vi "AlliGator Decay Actions.vi"(0 "AlliGator Q Elements in":T4[](array[typedef]), 1 "VI in":refnum<vi>, 2 "Script in":bool, 5 "AlliGator IV DVR in":refnum<data-value>, 7 "AlliGator Q Event in":T5=enum."GUI:Idle", 9 "Data":variant, 11 "error in (no error)":errorcluster, 12 "AlliGator Ctrl Refnums":T6) -> (3 "Script off":bool, 4 "AlliGator Q Elements out":T4[](array[typedef]), 6 "AlliGator IV DVR out":refnum<data-value>, 10 "[Notebook Message]":T1[](array[typedef]) {"Message Style"."Text Alignment" items=["Left", "Right", "Center"]}, 15 "error out":errorcluster)   [LabVIEW 2021, in "AlliGator Action Engine.lvlib"]
doc: "Processes AlliGator decay-related actions."
uses:
  AlliGator Action Engine.lvlib
  AlliGator Internal Variables v2.ctl
  <vilib>/vision/Image Controls.llb/IMAQ Image.ctl
  AlliGator Gate Image Set.ctl
  AlliGator FLI Dataset Type.ctl
  AlliGator Data Series Type.ctl
  AlliGator Dataset Channel.ctl
  AlliGator Gate Arithmetic.ctl
  AlliGator Displayed Image.ctl
  Image/Named ROI Description.ctl
  AlliGator Decay Metadata v3.ctl
  AlliGator Decay Background Subtraction Info.ctl
  AlliGator Baseline Subtraction Method.ctl
  Graphs/XY Graph/XY Graph Plot Shift Parameters.ctl
  Graphs/XY Graph/XY Graph Plot Shift Method.ctl
  AlliGator Decay Extrapolation Parameters.ctl
  Phasor/Calibration Phasor (m, phi).ctl
  Phasor/Phasor Reference Series.ctl
  Phasor/Phasor Calibration Map v2.ctl
  Phasor/Phasor (g, s).ctl
  AlliGator Raw Phasor Plot Data v4.ctl
  Phasor/Phasor Standard Deviation Options.ctl
  AlliGator Phasor Multi-Harmonic Data.ctl
  Phasor/Phasor Harmonic Data.ctl
  AlliGator Decay Fit Options & Parameters v2.ctl
  Fits/IRF(X)PSED/Decay Fit Options v2.ctl
  Fits/Decay Convolution/Decay Model.ctl
  Fits/Residual Type.ctl
  Fits/IRF(X)PSED/Fit Weights Type.ctl
  Fits/Non-linear Fitting Method v2.ctl
  Fits/Fit Calculation Method.ctl
  Fits/Non-linear Fitting Algorithm.ctl
  AlliGator Decay Fit Parameter Constraints 2.ctl
  Fits/IRF(X)PSED/Decay Fit Parameters In List.ctl
  Fits/IRF(X)PSED/MLE Baseline Offset Type.ctl
  AlliGator Decay Preprocessing Parameters.ctl
  Fits/IRF(X)PSED/Decay Fit Parameters & Derived Quantities List.ctl
  AlliGator Q Event.ctl
  AlliGator Ctrl Refnums.ctl
  AlliGator Other Ctrl Refnums.ctl
  AlliGator State Indicator.ctl
  AlliGator Phasor Plot Ctrl Refnums.ctl
  AlliGator Phasor Graph Ctrl Refnums.ctl
  Phasor/Phasor Calibration Type.ctl
  AlliGator Dataset Ctrl Refnums.ctl
  AlliGator Registered Events Ctrl Refnums.ctl
  AlliGator Image Histogram Control Refnums.ctl
  Histograms/Linear Histogram Options.ctl
  Histograms/Histogram Bin Option.ctl
  Histograms/Histogram Bin Position.ctl
  AlliGator Decay Fit Map Control Refnums.ctl
  AlliGator Q Element.ctl
  Notebook/Notebook Message Object.ctl
  Rich Text Box/Text Formatting.ctl
  Rich Text Box/Text Colors.ctl
  <vilib>/Utility/miscctls.llb/LVPoint32TypeDef.ctl
  Alligator Elements Order in Action Stack.ctl
  AlliGator State Indicators List.ctl
  AlliGator Settings List.ctl
  Graphs/XY Graph/XY Graph Selected Plot Info+Flag.ctl
  Graphs/XY Graph/XY Graph Refnum.ctl
  Fits/Square Pulse/Square Pulse Options.ctl
  Fits/Square Pulse/Square Pulse Levels Type.ctl
  Graphs/XY Graph/XY Graph Selected Plot Info.ctl
  Graphs/LabVIEW Plot Interpolation.ctl
  Variant/Variant to Data/Variant to I32.vi
  AlliGator Add Single Action to Stack.vi
  AlliGator Add Action Array to Stack.vi
  Variant/Variant to Data/Variant to U32.vi
  Variant/Variant to Data/Variant to DBL.vi
  GUI/GUI.lvlib
  AlliGator IRF.lvlib
  Variant/Variant to Data/Variant to Data.lvlib
  AlliGator GUI.lvlib
  AlliGator Decay Fit.lvlib
  Graphs/XY Graph/XY Graph Add-Ons.lvlib
  AlliGator Decay Processing.lvlib
  AlliGator Settings.lvlib
  Fits/Fits.lvlib
  AlliGator Internal Variables.lvlib
  AlliGator Decay Preprocessing.lvlib
  Graphs/Graphs.lvlib
  Sound/Sound.lvlib
  Fits/Abort Fit Global.vi
  AlliGator Intensity Corrections.lvlib
  Strings/Strings.lvlib
  Rich Text Box/Rich Text Box.lvlib
  Phasor/Phasor.lvlib
  Image/Image.lvlib
  AlliGator Phasor Graph.lvlib
  AlliGator Files.lvlib
  AlliGator Phasor Plot.lvlib
  AlliGator Source Image.lvlib
  AlliGator Decay Fit Parameter Map.lvlib
  AlliGator Dual-Channel Datasets.lvlib
  Histograms/Histogram Window.lvlib
  Notebook/Notebook.lvlib
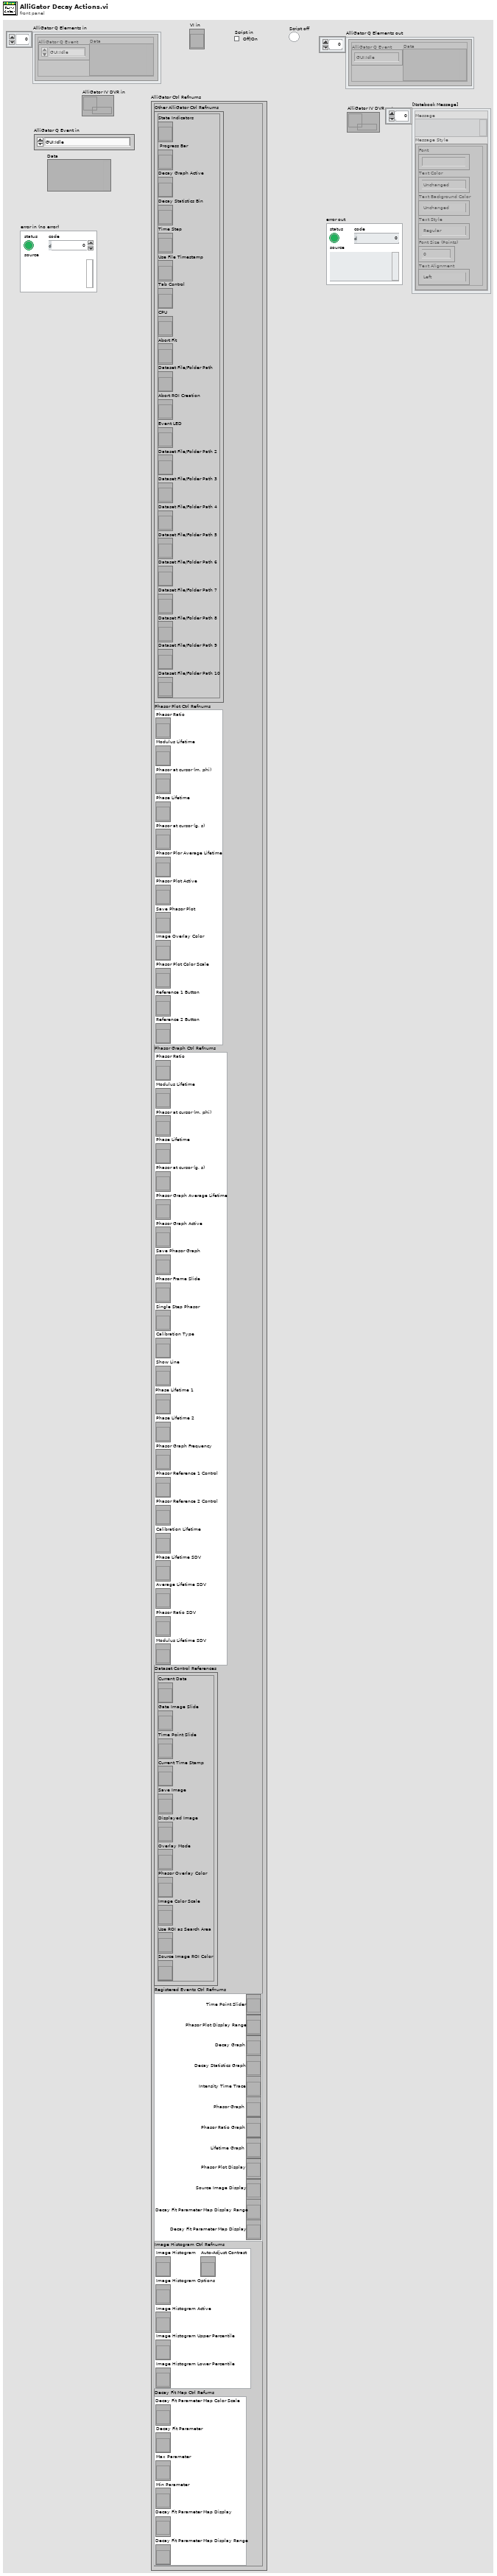
[diagram p1: front panel]
types:
  T1 = typedef "Notebook.lvlib/Notebook Message Object.ctl" = cluster{"Message":string, "Message Style":T2}
  T2 = typedef "Rich Text Box.lvlib/Text Formatting.ctl" = cluster{"Font":string, "Text Color":T3, "Text Background Color":T3, "Text Style":enum16{"Regular", "Bold", "Italic", "Underline", "Strikeout"}, "Font Size (Points)":dbl, "Text Alignment":i32}
  T3 = typedef "Rich Text Box.lvlib/Text Colors.ctl" = enum16{"Unchanged", "Black", "Blue", "Brown", "Gray", "Green", "Orange", "Pink", "Red", "White"}
  T4 = typedef "AlliGator Action Engine.lvlib/AlliGator Q Element.ctl" = cluster{"AlliGator Q Event":T5, "Data":variant}
  T5 = typedef "AlliGator Action Engine.lvlib/AlliGator Q Event.ctl" = enum16{"---- Files ----", "Files:Set Batch Export Files To Save", "Files:Set Dataset Loading & Pre-processing Options", "Files:Check #Frames in Dataset", "Files:Increment Frame Index", "Files:Open Mask Image", "Files:Open White Light Image", "Files:Open Single Dataset", "Files:New Folder of Folders Selected", "Files:Load File (all Types)_Scriptable", "Files:Move Flattened Series to Folders Series", "Files:Select Folder", "Files:Load FLI Dataset", "Files:Load Swiss SPAD 1 Dataset", "Files:Load Swiss SPAD 2 Dataset", "Files:Load .sdt FLI Dataset", "Files:Load .ptu FLI Dataset", "Files:Load .bin FLI Dataset", "Files:Load Single Gate Image Folder", "Files:Load I/m/phi Dataset (deprecated)", "Files:Load Single Image", "Files:Subtract Background File", "Files:Export FLI Dataset", "Files:Load HDF5 FLI Dataset", "Files:Set Destination File Path", "Files:Save Mask Image", "Files:Batch Conversion", "Files:New Folder Selected", "Files:Close FLI Dataset", "Files:Close FLI Dataset Series", "Files:Close White Light Image", "Files:Close Mask Image", "---- FLI Dataset ----", "FLI Dataset:Channel Arithmetic", "FLI Dataset:Export Average Lifetime Map as ASCII", "FLI Dataset:Export User-Defined Quantity Map as ASCII", "FLI Dataset:Python Function FLI Dataset Event", "FLI Dataset:ROI Analysis", "FLI Dataset:Tilted Logistic Square Gated IRF Characteristics Map", "FLI Dataset:Logistic Square Gated IRF Characteristics Map", "FLI Dataset:Square Gated IRF Characteristics Map", "FLI Dataset:Multi-ROI Single-Pixel Phasor Analysis", "FLI Dataset:Multi-ROI Single-Pixel NLSF Analysis", "FLI Dataset:All ROIs IRF Extraction", "FLI Dataset:All ROIs Decay Fit Non-Interactive (Fast + Individual IRF)", "FLI Dataset:All ROIs Phasor Analysis", "FLI Dataset:All ROIs Decay Fit", "FLI Dataset:Fluorescence Decay Statistics", "FLI Dataset:Update Decay Statistics Graph", "FLI Dataset:Get Decay from ROI", "FLI Dataset:All ROIs Average Lifetimes", "---- FLI Dataset Series ----", "FLI Dataset Series:Sum All Datasets in Series", "FLI Dataset Series:Add Dataset to Accumulated Dataset", "FLI Dataset Series:Display Accumulated Dataset", "FLI Dataset Series:Clear Dataset Series Sum", "FLI Dataset Series:Time-Series Analysis (NLSF)", "FLI Dataset Series:Time-Series Analysis (Phasor)", "---- Image ----", "Image:Update Image Profile Plots", "Image:Image Histogram Cursor Move", "Image:Image Histogram", "Image:Image Contrast", "Image:Set Image Histogram Cursor Move Flag", "Image:Clear Image Overlay", "Image:Use ROI as Search Area", "Image:Set ROI Diameter", "Image:Save Image Data as TIFF", "Image:Save Displayed Image with Overlay", "Image:Save Image Overlay Only", "Image:Save Image as Hot Pixel Mask", "Image:Change Source Image Color Palette", "Image:Copy Image to Clipboard", "Image:Source Image ROI Selection", "Image:Delete All ROIs", "Image:Delete All Unselected ROIs", "Image:Delete ROI", "Image:Merge All ROIs", "Image:Store ROI", "Image:Source Image ROI Storage", "Image:Export ROI Description to Notebook", "Image:Save ROI", "Image:Load ROI", "Image:Paste ROI Definition", "Image:Clear ROI", "Image:Identify ROIs in Mask Image", "Image:Create Complementary ROI", "Image:Create Contour ROI", "Image:Create ROI(s) from Pixels with Peak above Min_Scriptable", "Image:Create ROI(s) from Pixels with Intensity above Min_Scriptable", "Image:Compute ROI Statistics", "Image:Delete ROI(s) based on ROI Characteristics", "Image:Create ROI Grid", "Image:ROI to Individual Pixel ROIs", "Image:Python Function Source Image Event", "Image:Show Phasor Calibration Map ROI Centers", "Image:Convert ROI to Mask Image", "Image:Mouse Move", "Image:Mouse Up", "Image:Set Source Image Mouse Move Flag", "Image:Add Scale Bar Overlay", "Image:Delete Existing ROIs Option", "---- Decay ----", "Decay:Clear IRF/Reference Plot", "Decay:Clear Local IRFs", "Decay:Add Decay to Graph", "Decay:Smoothen Plot", "Decay:Smoothen Plot Tail", "Decay:Average Selected Plots", "Decay:Extract IRF", "Decay:Optimal IRF Extraction", "Decay:Threshold IRF", "Decay:Fit to Model IRF", "Decay:Fit IRF to Square Gate", "Decay:Fit IRF to Logistic Square Gate", "Decay:Fit IRF to Tilted Logistic Square Gate", "Decay:Create Bounding Cursors Set", "Decay:Export Bounding Cursors Definition to Notebook", "Decay:Denoise Plot", "Decay:Compute Cumulative Function", "Decay:Use as Reference Decay", "Decay:Show Reference Decay/IRF", "Decay:Extrapolate Decay", "Decay:Create Head & Tail Bounding Cursors", "Decay:Store Cursor-defined Head & Tail Fractions", "Decay:Rebin Plot", "Decay:1-Normalize Decay", "Decay:[0-1]-Normalize Plot", "Decay:Straighten Decay", "Decay:Shift Decay", "Decay:Fold Decay", "Decay:Fit Decay", "Decay:Global Fit of Selected Decays", "Decay:Post Global Fit Script", "Decay:Add Global Fit Parameters to Graph", "Decay:Add Decay Parameter(s) to Plot (Graph)", "Decay:Export Decay to Phasor Graph", "Decay:Plot Decay Shifts", "Decay:Compute Average Lifetime", "Decay:Plot Convolution", "Decay:Graph Tip Strip Update", "---- Decay Statistics ----", "Decay Statistics:Tip Strip Update", "---- Intensity Time Trace ----", "Intensity Time Trace:Use File Timestamp", "Intensity Time Trace:Load Intensity Corrections File", "Intensity Time Trace:Clear Intensity Corrections File", "Intensity Time Trace:Tip Strip Update", "---- Phasor Plot ----", "Phasor Plot:Build Phasor Plot", "Phasor Plot:Change Phasor Plot Color Palette", "Phasor Plot:Adjust Phasor Plot Display Range", "Phasor Plot:Highlight Image ROI in Phasor Plot", "Phasor Plot:Save Phasor Plot Image with Overlay", "Phasor Plot:Export Complex Phasor Map", "Phasor Plot:Export Phasor Ratio Map", "Phasor Plot:Export Average Lifetime Map", "Phasor Plot:Compute Phase Lifetime Histogram", "Phasor Plot:Compute Phasor Ratio Histogram", "Phasor Plot:Compute Phase Lifetime vs Intensity Scatter Plot", "Phasor Plot:Weber 2-Component Decomposition", "Phasor Plot:Update Phasor Color Map Vertices", "Phasor Plot:Clear Phasor Overlay", "Phasor Plot:Use Segment Extremities as References", "Phasor Plot:Use UC/Segment Intersections as References", "Phasor Plot:Use UC/Principal Axis Intersections as References", "Phasor Plot:Use UC/Linear Fit Intersections as References", "Phasor Plot:Update Phasor Plot Reference", "Phasor Plot:Show Local Phasor Info in Phasor Plot", "Phasor Plot:Update Phasor Plot State", "Phasor Plot:Phasor Plot ROI Storage", "Phasor Plot:Phasor Plot ROI Selection", "Phasor Plot:Python Function Phasor Plot Event", "Phasor Plot:Overlay Phasor ROI, Ratio or Map in Source Image", "Phasor Plot:Compute Decay of Selected Phasors", "Phasor Plot:Phasor at Image Pixel", "Phasor Plot:Mouse Move", "Phasor Plot:Mouse Up", "Phasor Plot:Display Range Mouse Move", "Phasor Plot:Set Mouse Move Flag", "---- Phasor Graph ----", "Phasor Graph:Calibrated Phasor Map Series", "Phasor Graph:Whole Image Phasor Scatter Plot (Todo)", "Phasor Graph:Get Phasor Value", "Phasor Graph:Create New Phasor Plot Dialog", "Phasor Graph:Update Last Phasor Value", "Phasor Graph:Update Phasor (m, phi)", "Phasor Graph:Remove Single Phasor from Plot", "Phasor Graph:Add Single Phasor to Plot", "Phasor Graph:Remove Phasor Plot", "Phasor Graph:Remove Selected Phasor Plots", "Phasor Graph:Clear Phasor Data", "Phasor Graph:Clear Phasor Graph", "Phasor Graph:Cursor Move", "Phasor Graph:Draw Cursor Connecting Line", "Phasor Graph:Clear Cursor Connecting Line", "Phasor Graph:Find UC Intersection", "Phasor Graph:Use UC/Cursor-Defined Line Intersections", "Phasor Graph:Use Selected Plots Fitted Line/UC Intersections", "Phasor Graph:Use Selected Plots Principal Axis/UC Intersections", "Phasor Graph:Show Single Phasor", "Phasor Graph:Save Single Phasor Plot", "Phasor Graph:Save All Phasor Plots", "Phasor Graph:Load Phasor Plot(s)", "Phasor Graph:Phasor Multiplication", "Phasor Graph:Compute Average Phasor", "Phasor Graph:Compute Multiple Average Phasors (Selected Plots)", "Phasor Graph:Export Single Phasor Plot Phase Lifetimes", "Phasor Graph:Phase Lifetime Trajectory", "Phasor Graph:Phase Lifetime vs Intensity Scatter Plot (deprecated)", "Phasor Graph:Parameter 2 vs Parameter 1 Scatter Plot", "Phasor Graph:Use Cursor n Location", "Phasor Graph:Set Reference n to Current Phase Lifetime Value", "Phasor Graph:Set Reference n to Lifetime Value", "Phasor Graph:Set Cursor n Location", "Phasor Graph:Save Phasor Graph Image", "Phasor Graph:Update SEPL Plot", "Phasor Graph:Export Single Phasor Plot Data", "Phasor Graph:Export Selected Phasor Plots Data", "Phasor Graph:Python Function Phasor Graph Event", "Phasor Graph:Tip Strip Update", "---- Calibration ----", "Calibration:Set Calibration Type", "Calibration:Load/Save Phasor Calibration", "Calibration:Load/Save Phasor Calibration Series", "Calibration:Load/Save Phasor Calibration Map", "Calibration:Use as Calibration", "Calibration:Compute Optimal Calibration from Phasor References", "Calibration:Clear Phasor Calibration", "Calibration:Single Phasor Calibration Information", "Calibration:Use as Calibration Series", "Calibration:Use as Calibration Map", "Calibration:Clear Calibration Series", "Calibration:Phasor Calibration Series Information", "Calibration:Clear Calibration Map", "Calibration:Phasor Calibration Map Information", "Calibration:Apply Phasor Calibration", "Calibration:Update Single Plot Calibration", "Calibration:Update Multiple Plots Calibration", "Calibration:Clear Single Plot Calibration", "Calibration:Clear All Plots Calibrations", "Calibration:Clear Plot(s) Calibration(s)?", "Calibration:Phasor Calibration Maps (# Gates Series)", "---- Phasor Ratio ----", "Phasor Ratio:Clear Reference n", "Phasor Ratio:Toggle Selected Plot(s)  Lock to Reference 1", "Phasor Ratio:Use as Reference n", "Phasor Ratio:Send Reference n to Notebook", "Phasor Ratio:Toggle Selected Plot(s)  Lock to Reference 2", "Phasor Ratio:Compute Phasor Ratio at Mouse Location", "Phasor Ratio:Compute Phasor Plot's Average Phasor Ratio", "Phasor Ratio:Compute Time-Series Phasor Ratios", "Phasor Ratio:Fit Line to Phasor Ratio Plot", "Phasor Ratio:Save References", "Phasor Ratio:Load References", "Phasor Ratio:Update Phasor Reference 1", "Phasor Ratio:Update Phasor Reference 2", "Phasor Ratio:Move Cursor n to Reference n", "Phasor Ratio:Use as Phasor Reference 1 Lifetime", "Phasor Ratio:Use as Phasor Reference 2 Lifetime", "Phasor Ratio:Export Phasor Ratio Map as ASCII", "Phasor Ratio:Tip Strip Update", "---- Lifetime & Other Parameters Graph ----", "Lifetime:Tip Strip Update", "---- Decay Fit Parameter Map ----", "Decay Fit Parameter Map:Export ROI NLSF Data as ASCII", "Decay Fit Parameter Map:Set Decay Fit  Parameter Map Selection", "Decay Fit Parameter Map:Build Decay Fit Parameter Map", "Decay Fit Parameter Map:Change Decay Fit Parameter Map Color Palette", "Decay Fit Parameter Map:Export Decay Fit Parameter Map Data as ASCII", "Decay Fit Parameter Map:Export All Decay Fit Parameter Maps Data as ASCII", "Decay Fit Parameter Map:Send Map Data to Lifetime Graph", "Decay Fit Parameter Map:Save Decay Fit Parameter Map Image", "Decay Fit Parameter Map:Save-Load IRFs & Fit Data", "Decay Fit Parameter Map:Update Local Decay Plots", "Decay Fit Parameter Map:Python Function Decay Fit Parameters Map Event", "Decay Fit Parameter Map:Overlay Decay Fit Parameter Map in Source Image", "Decay Fit Parameter Map:Plot Map Data vs Intensity", "Decay Fit Parameter Map:Mouse Up", "Decay Fit Parameter Map:Display Range Mouse Move", "---- Generic Graph ----", "Generic Graph:Generic XY Graph Event", "Generic Graph:Python Function XY Graph Event", "Generic Graph:New Plot", "Generic Graph:Save Plot", "Generic Graph:XY Plot Histogram", "Generic Graph:Set XY Graph Plot Name", "Generic Graph:Set Last Cursor Style", "Generic Graph:Tip Strip Update", "---- GUI ----", "GUI:Start Script", "GUI:Type of Displayed Image Changed", "GUI:Gate Image Slide Changed", "GUI:Show Busy Icon", "GUI:Show Busy Icon & Abort Button", "GUI:Hide Busy Icon", "GUI:Hide Busy Icon & Abort Button", "GUI:Abort", "GUI:End Script", "GUI:Start Timing", "GUI:End Timing", "GUI:Set State Indicator", "GUI:Send Parameters JSON Strings to Clipboard", "GUI:Set Gate Step", "GUI:Idle", "GUI:Initialization", "GUI:Quit", "GUI:Increment Dataset Index", "GUI:Set Dataset Index to -1", "GUI:Time Series Slider Moved", "GUI:Time Series Slider Changed", "GUI:Toggle Playback or Loop", "GUI:Playback Script", "GUI:Set Phasor Frequency", "GUI:Open Window", "GUI:Start Test Script", "GUI:End Test Script", "DEBUG"}
  T6 = typedef "AlliGator GUI.lvlib/AlliGator Ctrl Refnums.ctl" = cluster{"Other AlliGator Ctrl Refnums":T7, "Phasor Plot Ctrl Refnums":T8, "Phasor Graph Ctrl Refnums":T9, "Dataset Control References":T10, "Registered Events Ctrl Refnums":T11, "Image Histogram Ctrl Refnums":T12, "Decay Fit Map Ctrl Refums":T13}
  T7 = typedef "AlliGator GUI.lvlib/AlliGator Other Ctrl Refnums.ctl" = cluster{"State Indicators":refnum<vi>, " Progress Bar":refnum<vi>, "Decay Graph Active":refnum<vi>, "Decay Statistics Bin":refnum<vi>, "Time Step":refnum<vi>, "Use File Timestamp":refnum<vi>, "Tab Control":refnum<vi>, "CPU":refnum<vi>, "Abort Fit":refnum<vi>, "Dataset File/Folder Path":refnum<vi>, "Abort ROI Creation":refnum<vi>, "Event LED":refnum<vi>, "Dataset File/Folder Path 2":refnum<vi>, "Dataset File/Folder Path 3":refnum<vi>, "Dataset File/Folder Path 4":refnum<vi>, "Dataset File/Folder Path 5":refnum<vi>, "Dataset File/Folder Path 6":refnum<vi>, "Dataset File/Folder Path 7":refnum<vi>, "Dataset File/Folder Path 8":refnum<vi>, "Dataset File/Folder Path 9":refnum<vi>, "Dataset File/Folder Path 10":refnum<vi>}
  T8 = typedef "AlliGator GUI.lvlib/AlliGator Phasor Plot Ctrl Refnums.ctl" = cluster{"Phasor Ratio":refnum<vi>, "Modulus Lifetime":refnum<vi>, "Phasor at cursor (m, phi)":refnum<vi>, "Phase Lifetime":refnum<vi>, "Phasor at cursor (g, s)":refnum<vi>, "Phasor Plor Average Lifetime":refnum<vi>, "Phasor Plot Active":refnum<vi>, "Save Phasor Plot":refnum<vi>, "Image Overlay Color":refnum<vi>, "Phasor Plot Color Scale":refnum<vi>, "Reference 1 Button":refnum<vi>, "Reference 2 Button":refnum<vi>}
  T9 = typedef "AlliGator GUI.lvlib/AlliGator Phasor Graph Ctrl Refnums.ctl" = cluster{"Phasor Ratio":refnum<vi>, "Modulus Lifetime":refnum<vi>, "Phasor at cursor (m, phi)":refnum<vi>, "Phase Lifetime":refnum<vi>, "Phasor at cursor (g, s)":refnum<vi>, "Phasor Graph Average Lifetime":refnum<vi>, "Phasor Graph Active":refnum<vi>, "Save Phasor Graph":refnum<vi>, "Phasor Frame Slide":refnum<vi>, "Single Step Phasor":refnum<vi>, "Calibration Type":refnum<vi>, "Show Line":refnum<vi>, "Phase Lifetime 1":refnum<vi>, "Phase Lifetime 2":refnum<vi>, "Phasor Graph Frequency":refnum<vi>, "Phasor Reference 1 Control":refnum<vi>, "Phasor Reference 2 Control":refnum<vi>, "Calibration Lifetime":refnum<vi>, "Phase Lifetime SDV":refnum<vi>, "Average Lifetime SDV":refnum<vi>, "Phasor Ratio SDV":refnum<vi>, "Modulus Lifetime SDV":refnum<vi>}
  T10 = typedef "AlliGator GUI.lvlib/AlliGator Dataset Ctrl Refnums.ctl" = cluster{"Current Data":refnum<vi>, "Gate Image Slide":refnum<vi>, "Time Point Slide":refnum<vi>, "Current Time Stamp":refnum<vi>, "Save Image":refnum<vi>, "Displayed Image":refnum<vi>, "Overlay Mode":refnum<vi>, "Phasor Overlay Color":refnum<vi>, "Image Color Scale":refnum<vi>, "Use ROI as Search Area":refnum<vi>, "Source Image ROI Color":refnum<vi>}
  T11 = typedef "AlliGator GUI.lvlib/AlliGator Registered Events Ctrl Refnums.ctl" = cluster{"Time Point Slider":refnum<vi>, "Phasor Plot Display Range":refnum<vi>, "Decay Graph":refnum<vi>, "Decay Statistics Graph":refnum<vi>, "Intensity Time Trace":refnum<vi>, "Phasor Graph":refnum<vi>, "Phasor Ratio Graph":refnum<vi>, "Lifetime Graph":refnum<vi>, "Phasor Plot Display":refnum<vi>, "Source Image Display":refnum<vi>, "Decay Fit Parameter Map Display Range":refnum<vi>, "Decay Fit Parameter Map Display":refnum<vi>}
  T12 = typedef "AlliGator GUI.lvlib/AlliGator Image Histogram Control Refnums.ctl" = cluster{"Image Histogram":refnum<vi>, "Image Histogram Options":refnum<vi>, "Image Histogram Active":refnum<vi>, "Image Histogram Upper Percentile":refnum<vi>, "Image Histogram Lower Percentile":refnum<vi>, "Auto-Adjust Contrast":refnum<vi>}
  T13 = typedef "AlliGator Decay Fit Parameter Map.lvlib/AlliGator Decay Fit Map Control Refnums.ctl" = cluster{"Decay Fit Parameter Map Color Scale":refnum<vi>, "Decay Fit Parameter":refnum<vi>, "Max Parameter":refnum<vi>, "Min Parameter":refnum<vi>, "Decay Fit Parameter Map Display":refnum<vi>, "Decay Fit Parameter Map Display Range":refnum<vi>}
  T14 = typedef "AlliGator Action Engine.lvlib/Alligator Elements Order in Action Stack.ctl" = enum16{"Enqueue 2 AFTER 1", "Enqueue 2 BEFORE 1"}
  T15 = typedef "AlliGator Action Engine.lvlib/AlliGator State Indicators List.ctl" = enum16{"Phasor Calibration Defined", "Phasor Calibration Series Defined", "Phasor Calibration Map Defined", "Phasor Reference 1 Defined", "Phasor Reference 2 Defined", "Lifetime Reference 1 Defined", "Lifetime Reference 2 Defined", "Phasor Calibration Used", "Phasor Calibration Series Used", "Phasor Calibration Map Used", "Dataset Update Needed", "Phasor Plot Update Needed", "Reference/IRF Defined", "Individual IRFs Defined"}
  T16 = typedef "AlliGator Settings.lvlib/AlliGator Settings List.ctl" = enum16{"GUI:Visible Settings Tab", "GUI:Last Run Version", "Source Image:Use Image Histogram for Contrast", "Source Image:Low Count Pixels Rejection Options", "Source Image:High Count Pixels Rejection Options", "Source Image:Use Image Brightness", "Source Image:Blend Overlay with Image Background", "Source Image:Use Fixed ROI Diameter", "Source Image:ROI Diameter", "Source Image:ROI Center Color", "Source Image:Peak Threshold", "Source Image:Intensity Threshold", "Source Image:Image Binning Options", "Source Image:Image Smoothing Options", "Source Image:Image Histogram Active", "Source Image:Invert Binary Mask", "Source Image:Hot Pixel Removal", "Source Image:Overlay Analyzed ROI Center", "Source Image:Auto-Adjust Contrast", "Source Image:Histogram Lower Percentile", "Source Image:Histogram Upper Percentile", "Source Image:Save Source Image", "Source Image:Scale Bar Options", "Source Image:Image Resolution (Pixel Size)", "Source Image:Flatfield Correction", "Source Image:Show Dead Left Columns Correction", "Source Image:Dead Left Columns Correction", "Source Image:Image Pre-Processing Operations Order", "Data Information:Gate Width", "Data Information:Nanotime Gate Separation", "Data Information:Macrotime Gate Separation", "Data Information:Gate Step", "Data Information:# Gates", "Data Information:Gate Image Exposure", "Data Information:Gate Image Integration", "Data Information:Gates to Skip", "Data Information:Gates to Keep", "Data Information:Define Gates to", "Data Information:Channel Name", "Data Information:Available Channel Names", "Data Information:Channel Arithmetic", "Data Information:Background File Subtraction", "Data Information:Background File", "Data Information:Background Scaling Factor", "Data Information:Background Pile-up Correction", "Data Information:Background Pixel Well Capacity", "Data Information:Laser Period", "Data Information:SYNC Period", "Data Information:Pile-up Correction", "Data Information:Pixel Well Capacity", "Data Information:Dataset Scaling Factor", "Fluorescence Decay_Decay Pre-Processing:Reverse Gates", "Fluorescence Decay_Decay Pre-Processing:Verbose Decay Pre-Processing", "Fluorescence Decay_Decay Pre-Processing:Use Decay Pre-Processing", "Fluorescence Decay_Decay Pre-Processing:Background Subtraction", "Fluorescence Decay_Decay Pre-Processing:Background Definition Range", "Fluorescence Decay_Decay Pre-Processing:Baseline Subtraction Method", "Fluorescence Decay_Decay Pre-Processing:Decay Pre-Processing Operations Order", "Fluorescence Decay_Decay Pre-Processing:Smoothing Parameter", "Fluorescence Decay_Decay Pre-Processing:Shift Decay", "Fluorescence Decay_Decay Pre-Processing:Decay Shift Parameters", "Fluorescence Decay_Decay Pre-Processing:Fold Decay", "Fluorescence Decay_Decay Pre-Processing:# Folds", "Fluorescence Decay_Decay Pre-Processing:1-Normalize Decay", "Fluorescence Decay_Decay Pre-Processing:[0-1]-Normalize Decay", "Fluorescence Decay_Decay Pre-Processing:Smoothen Decay", "Fluorescence Decay_Decay Pre-Processing:Extrapolate Decay", "Fluorescence Decay_Decay Pre-Processing:Use Periodicity", "Fluorescence Decay_Decay Pre-Processing:Use Cursors", "Fluorescence Decay_Decay Pre-Processing:Tail Fraction", "Fluorescence Decay_Decay Pre-Processing:Head Fraction", "Fluorescence Decay_Decay Pre-Processing:Additional Points", "Fluorescence Decay_Decay Pre-Processing:Straighten Decay", "Fluorescence Decay_Decay Pre-Processing:Constant Background", "Fluorescence Decay_Decay Pre-Processing:Pixel-Normalize Decay", "Fluorescence Decay_Advanced Analysis:Extract IRF instead of Decay", "Fluorescence Decay_Advanced Analysis:IRF Extraction Options", "Fluorescence Decay_Advanced Analysis:IRF Optimization Options", "Fluorescence Decay_Advanced Analysis:Square Pulse Options", "Fluorescence Decay_Advanced Analysis:IRF Order", "Fluorescence Decay_Advanced Analysis:IRF Time Constants", "Fluorescence Decay_Advanced Analysis:Wavelet Analysis Options", "Fluorescence Decay_Advanced Analysis:Average Lifetime Options", "Fluorescence Decay_Fit Options:Fit Options", "Fluorescence Decay_Fit Options:Use Legacy Fitting Approach", "Fluorescence Decay_Fit Options:Use Data Information Laser Period", "Fluorescence Decay_Fit Parameters:Displayed Fit Parameters", "Fluorescence Decay_Fit Parameters:Fit Parameter Constraints", "Fluorescence Decay_Fit Parameters:Export Tabulated Results", "Fluorescence Decay_Fit Parameters:MLE Baseline Offset Type", "Fluorescence Decay_Fit Parameters:MLE Baseline Offset", "Fluorescence Decay_Fit Parameters:Guess Parameter Names", "Fluorescence Decay_Fit Parameters:Guess Parameter Values", "Fluorescence Decay_Fit Parameters:Guess Parameters Options", "Fluorescence Decay_Styles:Show Last Decay Only", "Fluorescence Decay_Styles:Decay Graph Color Array", "Fluorescence Decay:Decay Graph Active", "Fluorescence Decay Statistics:Min Peak Value", "Fluorescence Decay Statistics:Reject Low Decay Peak Pixels", "Fluorescence Decay Statistics:Reject High Decay Peak Pixels", "Fluorescence Decay Statistics:Max Peak Value", "Time Traces:Use File Timestamp", "Time Traces:Time Step", "Time Traces:Use Intensity Correction File", "Time Traces:Intensity Correction File", "Phasor Plot:Phasor Plot Smoothing Options", "Phasor Plot:Phasor Plot Size", "Phasor Plot:Phasor Plot Graphics Options", "Phasor Plot:Cumulative Phasor Plot", "Phasor Plot:Use Phasor Brightness", "Phasor Plot:Blend Overlay with Phasor Background", "Phasor Plot:Save Phasor Plot", "Phasor Plot:Show References", "Phasor Plot:Phasor Ratio Decay Range", "Phasor Plot:Exponential Fading", "Phasor Plot:Phasor Ratio Reference Colors", "Phasor Plot:Reference Radius", "Phasor Plot:Show Color Map Vertices", "Phasor Plot:Phasor Plot Active", "Phasor Plot:Phasor Ratio Color Map Type", "Phasor Plot:Phasor Ratio Color Map", "Phasor Plot:Phasor Ratio Display Range", "Phasor Plot:Selected Image ROI(s)", "Phasor Plot:All Image ROIs", "Phasor Plot:Selected Phasor Plot ROI(s)", "Phasor Plot:All Phasor Plot ROIs", "Phasor Plot:Phasor Ratio Color-Coded Quantity", "Phasor Plot:Store Phasor Harmonics", "Phasor Plot:Draw Reference Segment", "Phasor Plot:User-Defined Quantity", "Phasor Graph:Phasor Frequency", "Phasor Graph:Phasor Ratio Type", "Phasor Graph:Pixel-level Phasor Computation", "Phasor Graph:Save Phasor Graph", "Phasor Graph:Phasor Graph Active", "Phasor Graph:Phasor SDV Options", "Phasor Calibration:Use Backup Calibration if needed", "Phasor Graph:Define Shortest Lifetime as", "Phasor Calibration:Backup Calibration Type", "Phasor Calibration:Calibration Type", "Phasor Calibration:Calibration Lifetime", "Phasor Calibration:Calibration Map Algorithm", "Single-Exponential Phasor Locus (SEPL):Gate Parameters", "Single-Exponential Phasor Locus (SEPL):User-defined Gate", "Single-Exponential Phasor Locus (SEPL):User-defined IRF", "Single-Exponential Phasor Locus (SEPL):Phasor Parameters", "Single-Exponential Phasor Locus (SEPL):Decay & IRF Parameters", "Single-Exponential Phasor Locus (SEPL):Display Parameters", "Lifetime Analysis:Decay Analysis Parameters", "Lifetime Analysis:Lifetime Map Active", "Plugins:Python Settings", "Miscellaneous:Verbose Mode", "Miscellaneous:Beep after Script", "Miscellaneous:Saved Image File Format", "Miscellaneous:Exported Gate Image Settings", "Miscellaneous:Include Loading in Timing", "Miscellaneous:Verbose Settings Mode", "Miscellaneous:Histogram Options", "Miscellaneous:Beep on Error", "Miscellaneous:# Logical Processors Used", "Miscellaneous:ROI Description Max Characters", "Miscellaneous:Verbose Error Mode", "Miscellaneous:Transparent Mask Color"}
  T17 = typedef "XY Graph Add-Ons.lvlib/XY Graph Selected Plot Info+Flag.ctl" = cluster{"Multiplot XY Graph":T18, "Mouse Coordinates":T19, "Plot Index":i32, "Flag":bool}
  T18 = typedef "XY Graph Add-Ons.lvlib/XY Graph Refnum.ctl" = refnum<vi>
  T19 = typedef "LVPoint32TypeDef.ctl" = cluster{"Horizontal":i32, "Vertical":i32}
  T20 = typedef "Fits.lvlib/Square Pulse Options.ctl" = cluster{"Method":T21, "# Bins":i32, "Threshold %":dbl, "Center on Midpoint":bool, "Smoothen Plot":bool}
  T21 = typedef "Fits.lvlib/Square Pulse Levels Type.ctl" = enum16{"Mode", "Mean"}
  T22 = typedef "XY Graph Add-Ons.lvlib/XY Graph Selected Plot Info.ctl" = cluster{"Multiplot XY Graph":T18, "Mouse Coordinates":T19, "Plot Index":i32}
  T23 = typedef "AlliGator Decay Analysis.lvlib/AlliGator Decay Fit.lvlib/AlliGator Decay Fit Output Options.ctl" = cluster{"Fit Model":T24, "Decay Fit Parameter Array":T25[]}
  T24 = typedef "Fits.lvlib/Decay Model.ctl" = enum16{"1-Exponential", "2-Exponentials"}
  T25 = typedef "Fits.lvlib/Decay Fit Parameters & Derived Quantities List.ctl" = enum16{"Offset", "Baseline", "A_1", "tau_1", "A_2", "tau_2", "<tau>_a", "f1_a", "f2_a", "<tau>_i", "f1_i", "f2_i", "-", "R^2", "Chi^2"}
  T26 = cluster{"CtlRef":refnum<vi>, "Coords":T19, "Plot ID":i32}
  T27 = typedef "Math.lvlib/Wavelet Analysis Options.ctl" = cluster{"Wavelet":enum16{"db02", "db03", "db04", "db05", "db06", "db07", "db08", "db09", "db10", "db11", "db12", "db13", "db14", "Haar", "bior1_3", "bior1_5", "bior2_2", "bior2_4", "bior2_6", "bior2_8", "bior3_1", "bior3_3", "bior3_5", "bior3_7", "bior3_9", "bior4_4 (FBI)", "bior5_5", "bior6_8", "coif1", "coif2", "coif3", "coif4", "coif5", "sym2", "sym3", "sym4", "sym5", "sym6", "sym7", "sym8"}, "Option for Approximate Coefficients":enum16{"None", "Threshold", "Detrend"}, "# Levels":i32, "Threshold Settings":cluster{"Thresholding Rule":enum16{"SURE", "Hybrid", "Universal", "Minimax"}, "Rescaling Method":enum16{"One", "Single level", "Multiple levels"}, "Soft Threshold?":bool}, "Wavelet Transform Type":enum16{"Discrete", "Undecimated"}}
  T28 = typedef "ROI Descriptor" = cluster{"Global Rectangle":i32[], "Contours":cluster{"ID":enum32{"External", "Internal"}, "Type":u32, "Coordinates":i32[]}[]}
  T29 = typedef "XY Graph Add-Ons.lvlib/XY Plot Data.ctl" = cluster{"X Array":dbl[], "Y Array":dbl[]}
  T30 = typedef "AlliGator Decay Fit Parameter Map.lvlib/AlliGator Decay Fit Options & Parameters v2.ctl" = cluster{"SYNC Period":dbl[unit], "Fit Options":T31, "Fit Parameter Constraints":T37[], "MLE Baseline Offset":dbl, "MLE Baseline Offset Type":T39}
  T31 = typedef "Fits.lvlib/Decay Fit Options v2.ctl" = cluster{"Show Fit Residuals":bool, "Fit Model":T24, "Residual Type":T32, "Max Decay Percentile":dbl, "Min Decay Percentile":dbl, "Show Full Decay":bool, "Weights":T33, "Fitting Method":T34, "Compute Parameter Uncertainties":bool, "Periodic Boundaries":bool, "Model Calculation":T35, "Period":dbl[unit], "Termination Criteria":cluster{"Max Iterations":i32, "Max Function Calls":i32, "Max Time":dbl[unit], "Function Tolerance":dbl, "Parameter Tolerance":dbl, "Gradient Tolerance":dbl, "Min Lambda":dbl, "Max Lambda":dbl, "Initial Tick Count":u32}, "Offset Resolution":dbl[unit], "Use Local IRF":bool, "Fitting Algorithm":T36}
  T32 = typedef "Fits.lvlib/Residual Type.ctl" = enum16{"Standard", "Normalized", "Reduced"}
  T33 = typedef "Fits.lvlib/Fit Weights Type.ctl" = enum16{"Unweighted", "1/Variance", "Best of All"}
  T34 = typedef "Fits.lvlib/Non-linear Fitting Method v2.ctl" = enum16{"Least Square", "Least Absolute Residual", "Bisquare", "MLE", "-", "Best of All"}
  T35 = typedef "Fits.lvlib/Fit Calculation Method.ctl" = enum16{"Simulation", "Convolution", "Integration"}
  T36 = typedef "Fits.lvlib/Non-linear Fitting Algorithm.ctl" = enum16{"Levenberg-Marquardt", "Trust-Region Dogleg"}
  T37 = typedef "AlliGator Decay Analysis.lvlib/AlliGator Decay Fit.lvlib/AlliGator Decay Fit Parameter Constraints 2.ctl" = cluster{"Fit Parameter":T38, "Min Value":dbl, "Max Value":dbl, "Global":bool, "Used":bool}
  T38 = typedef "Fits.lvlib/Decay Fit Parameters In List.ctl" = enum16{"Offset", "Baseline", "A_1", "tau_1", "A_2", "tau_2"}
  T39 = typedef "Fits.lvlib/MLE Baseline Offset Type.ctl" = enum32{"Absolute", "Percentage"}
  T40 = cluster{"t Array":dbl[], "Amplitude Array":dbl[]}
  T41 = typedef "XY Graph Add-Ons.lvlib/XY Graph Plot Shift Parameters.ctl" = cluster{"Type":T42, "Shift":dbl[unit], "Threshold":dbl, "Rotate":bool}
  T42 = typedef "XY Graph Add-Ons.lvlib/XY Graph Plot Shift Method.ctl" = enum16{"Default", "CFD", "Threshold", "Cross-Correlation"}
  T43 = typedef "Graphs.lvlib/LabVIEW Plot Interpolation.ctl" = u8
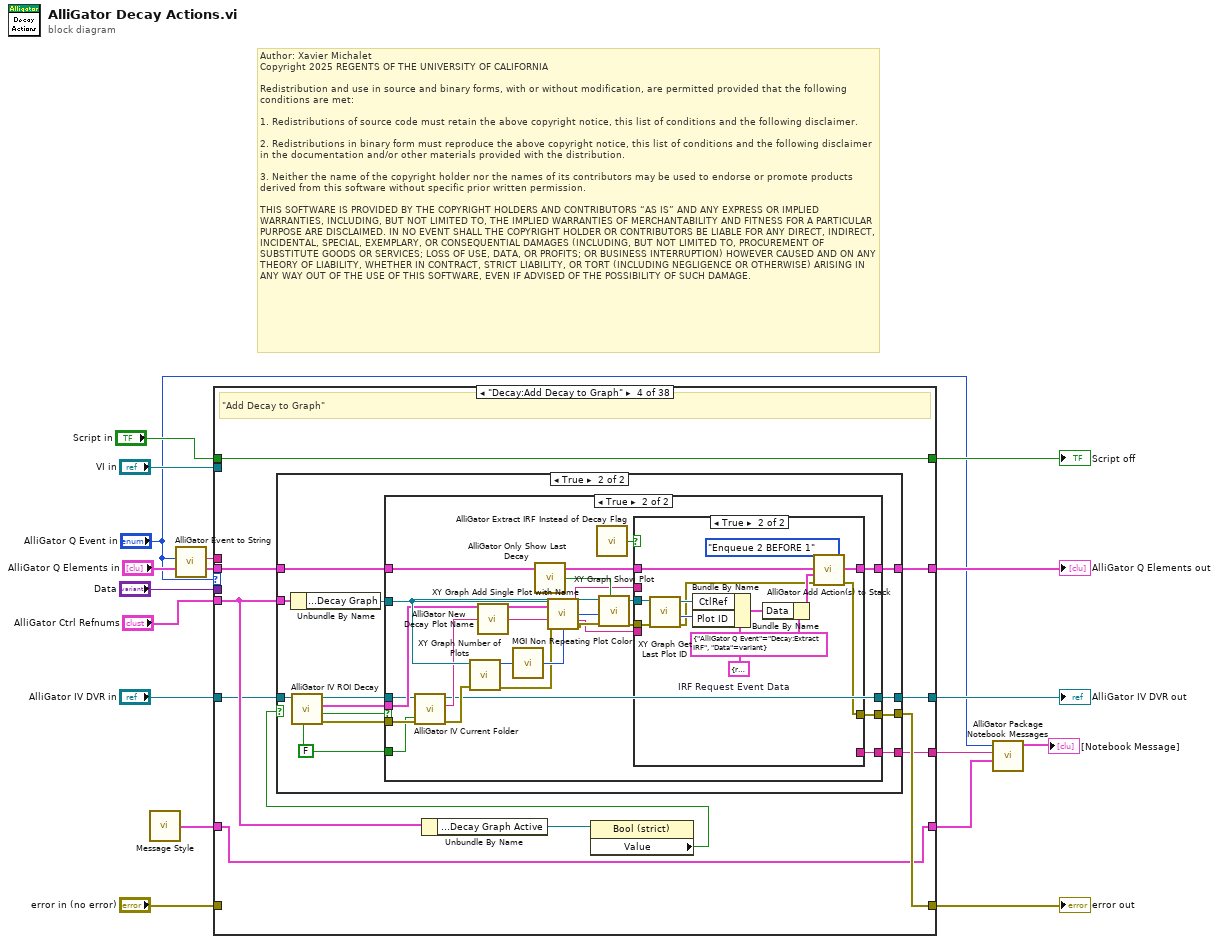
[diagram p0: block diagram]
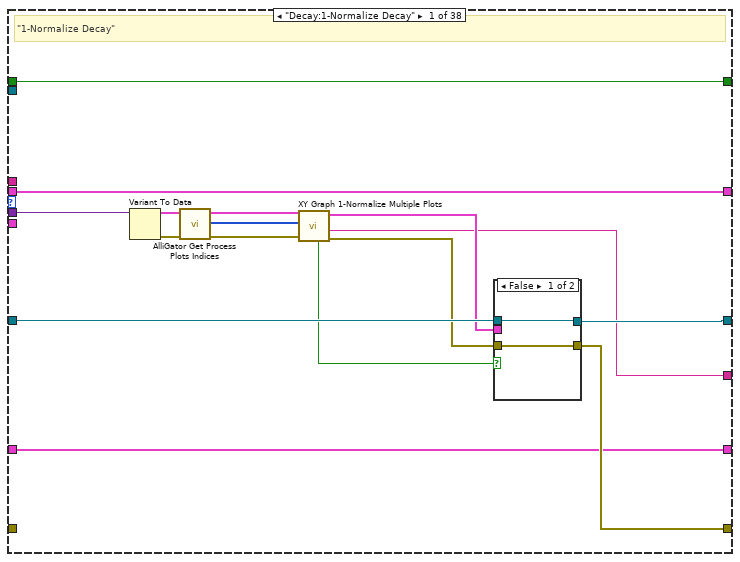
[diagram p2: hidden frame]
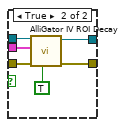
[diagram p3: hidden frame]
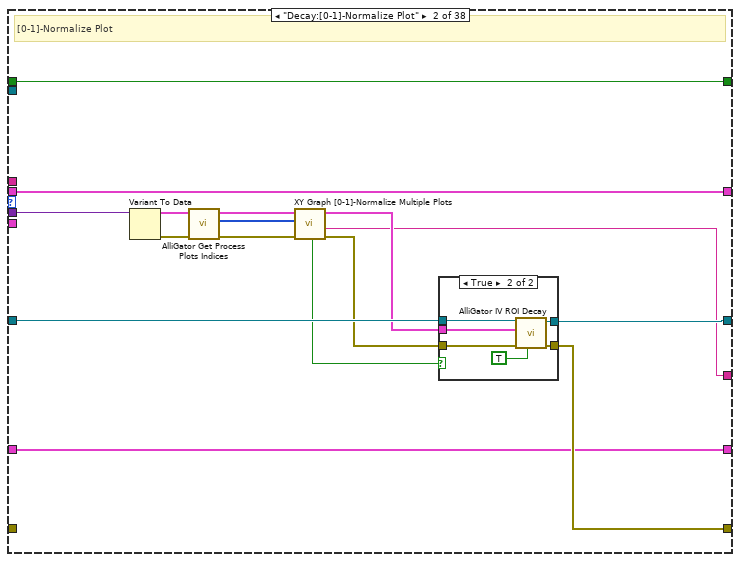
[diagram p4: hidden frame]
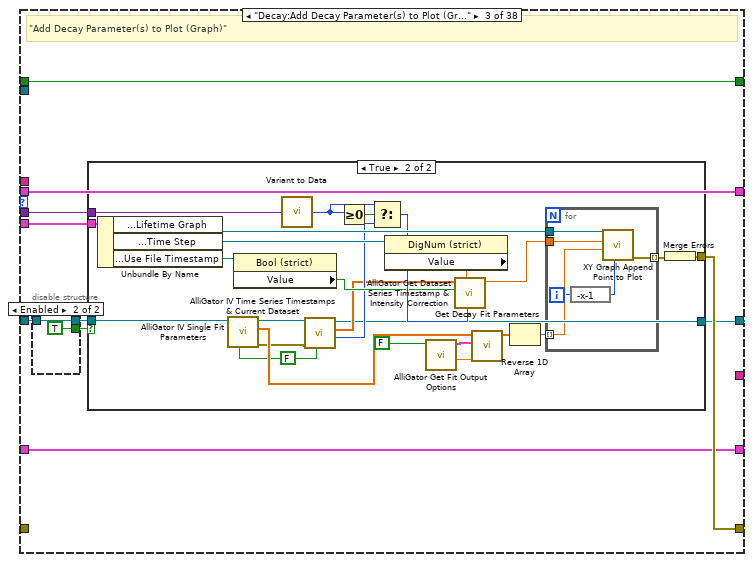
[diagram p6: hidden frame]
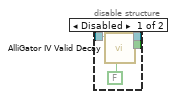
[diagram p7: hidden frame]
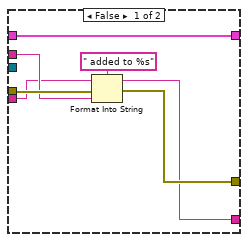
[diagram p11: hidden frame]
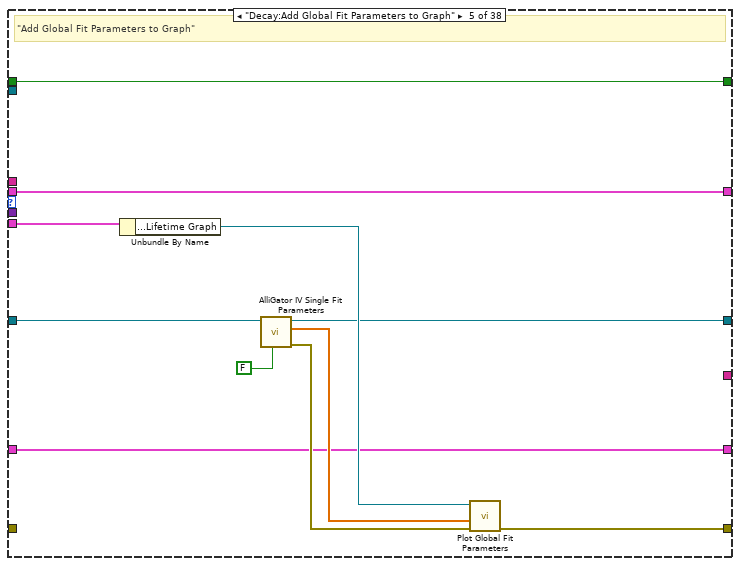
[diagram p12: hidden frame]
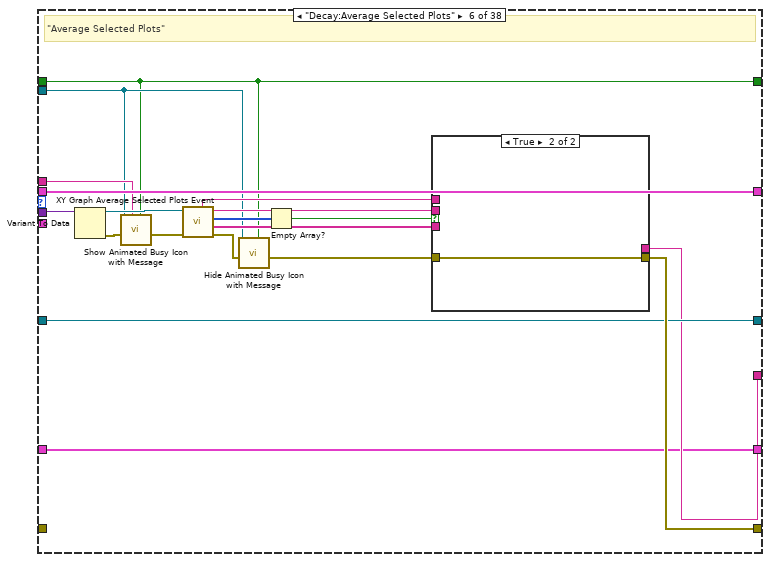
[diagram p13: hidden frame]
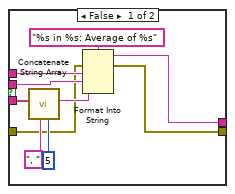
[diagram p14: hidden frame]
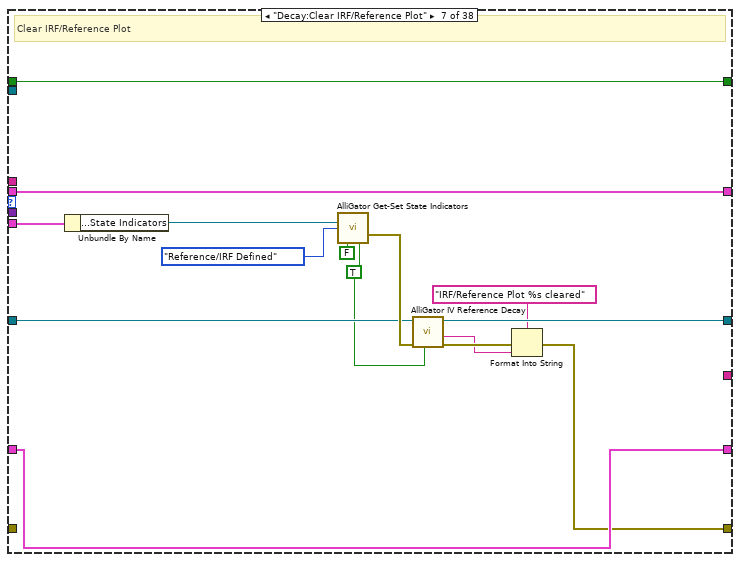
[diagram p15: hidden frame]
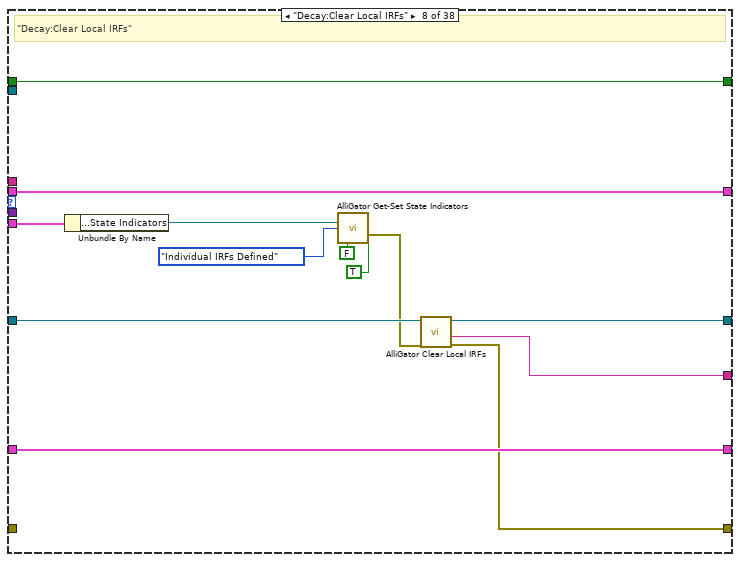
[diagram p16: hidden frame]
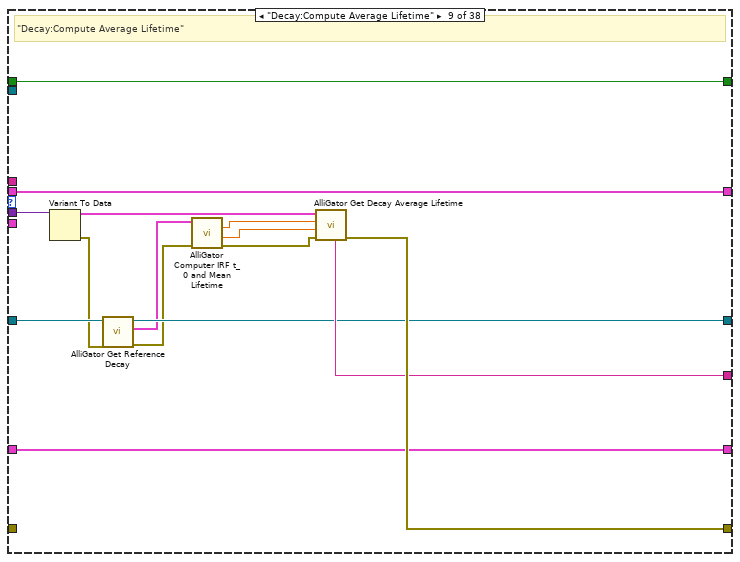
[diagram p17: hidden frame]
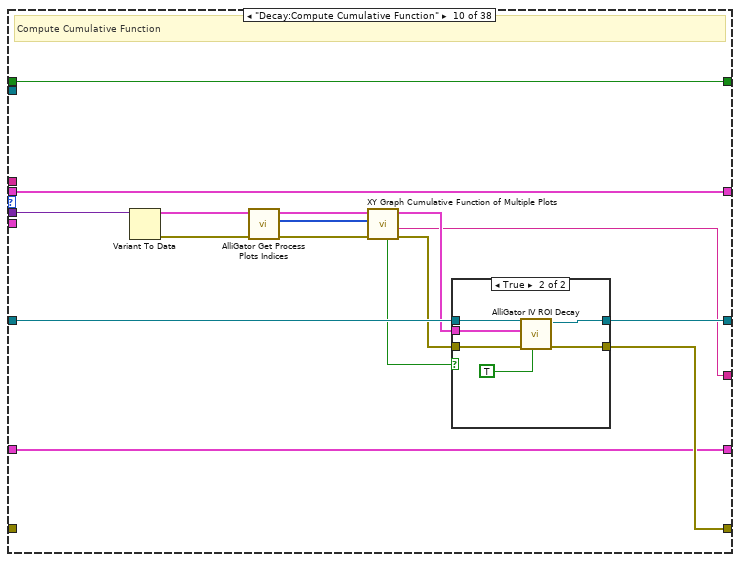
[diagram p18: hidden frame]
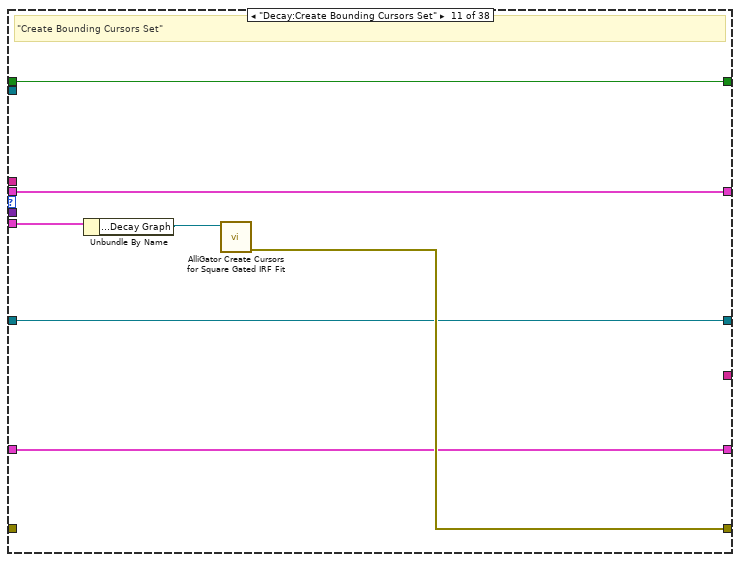
[diagram p20: hidden frame]
diagram:
  # "Author: Xavier Michalet\nCopyright 2025 REGENTS OF THE UNIVERSITY OF CALIFORNIA\n\nRedistribution and use in source and binary forms, with or without modification, are permitted provided that the following conditions are met:\n\n1. Redistributions of source code must retain the above copyright notice, this list of conditions and the following disclaimer.\n\n2. Redistributions in binary form must reproduce the above copyright notice, this list of conditions and the following disclaimer in the documentation and/or other materials provided with the distribution.\n\n3. Neither the name of the copyright holder nor the names of its contributors may be used to endorse or promote products derived from this software without specific prior written permission.\n\nTHIS SOFTWARE IS PROVIDED BY THE COPYRIGHT HOLDERS AND CONTRIBUTORS “AS IS” AND ANY EXPRESS OR IMPLIED WARRANTIES, INCLUDING, BUT NOT LIMITED TO, THE IMPLIED WARRANTIES OF MERCHANTABILITY AND FITNESS FOR A PARTICULAR PURPOSE ARE DISCLAIMED. IN NO EVENT SHALL THE COPYRIGHT HOLDER OR CONTRIBUTORS BE LIABLE FOR ANY DIRECT, INDIRECT, INCIDENTAL, SPECIAL, EXEMPLARY, OR CONSEQUENTIAL DAMAGES (INCLUDING, BUT NOT LIMITED TO, PROCUREMENT OF SUBSTITUTE GOODS OR SERVICES; LOSS OF USE, DATA, OR PROFITS; OR BUSINESS INTERRUPTION) HOWEVER CAUSED AND ON ANY THEORY OF LIABILITY, WHETHER IN CONTRACT, STRICT LIABILITY, OR TORT (INCLUDING NEGLIGENCE OR OTHERWISE) ARISING IN ANY WAY OUT OF THE USE OF THIS SOFTWARE, EVEN IF ADVISED OF THE POSSIBILITY OF SUCH DAMAGE."
  n1 = call "Message Style.vi"() -> ("Message Formatting"=w5:T2)
  n2 = call "AlliGator Event to String.vi"("AlliGator Q Event"="AlliGator Q Event in") -> ("String"=w8:string)  [unwired: 8 in]
  n3 = case shown="\"Decay:Add Decay to Graph\"" "AlliGator Q Event in" {
    selector: "AlliGator Q Event in" -> [_ _ _ _ _ _ _ _ _ _ _ _ _ _ _ _ _ _ _ _ _ _ _ _ _ w678 _ _ _ _ _ _ _ _ _ _ w918 _]
    tunnel: "Data" -> [w32 w56 w72 _ _ w217 _ _ w268 w286 _ _ w330 _ w351 w400 w416 w436 w478 w515 w532 w549 w568 _ w656 w680 _ _ w731 w766 _ w815 w844 w859 w877 w898 w920 _]
    tunnel: "AlliGator Q Elements in" -> [w33 w57 w75 w125 w198 w216 w243 w256 w271 w287 w302 w309 w331 w350 w361 w401 w417 w437 w484 w516 w533 w550 w569 w587 w657 w681 w705 w713 w732 w767 w787 w816 w845 w862 w878 w899 w921 w926]
    tunnel: [w33 w57 w75 w124 w198 w216 w243 w256 w271 w287 w302 w309 w331 w350 w360 w401 w417 w437 w484 w516 w533 w550 w569 w586 w657 w681 w705 w712 w732 w767 w787 w816 w845 w862 w878 w899 w921 w926] -> w10
    tunnel: "VI in" -> [_ _ _ _ _ w203 _ _ _ _ _ _ _ _ _ w394 _ w432 w486 w504 w528 w545 _ w583 w650 _ _ _ _ _ _ _ _ _ _ _ _ _]
    tunnel: [w30 w54 w74 w123 w197 w199 w242 w255 w270 w284 w301 w308 w322 w342 w362 w385 w414 w434 w476 w493 w517 w534 w567 w585 w641 w676 w700 w716 w729 w765 w786 w810 w839 w861 w875 w896 w916 w925] -> w7
    tunnel: "Script in" -> [w30 w54 w74 w123 w197 w199 w242 w255 w270 w284 w301 w308 w322 w342 w362 w385 w414 w434 w476 w493 w517 w534 w567 w585 w641 w676 w700 w716 w729 w765 w786 w810 w839 w861 w875 w896 w916 w925]
    tunnel: w8 -> [_ _ _ _ _ w204 _ _ _ _ _ _ _ _ _ w395 _ w433 w485 w503 w527 w544 _ w582 w651 _ _ _ _ _ _ _ _ _ _ _ _ _]
    tunnel: "error in (no error)" -> [_ _ _ _ _ _ _ _ _ _ _ _ _ _ _ _ _ _ _ _ _ _ _ _ _ _ _ _ _ _ _ _ _ _ _ _ _ w924]
    tunnel: [w26 w50 w73 w122 w196 w205 w231 w245 w269 w279 w300 w307 w319 w345 w359 w390 w409 w435 w481 w498 w523 w539 w561 w588 w646 w677 w701 w709 w724 w762 w785 w806 w835 w860 w870 w891 w917 w924] -> w6
    tunnel: "AlliGator Ctrl Refnums" -> [_ _ w71 w120 w194 _ w241 w254 _ _ w298 w305 _ w344 w357 _ _ _ _ _ _ _ _ w584 _ _ w698 w714 _ _ w780 _ _ _ _ _ w914 _]
    tunnel: "AlliGator IV DVR in" -> [w28 w52 w67 w118 w193 w202 w235 w248 w262 w283 w297 w304 w317 w343 w355 w393 w413 w427 w483 w501 w525 w543 w563 w581 w649 w673 w696 w707 w727 w761 w779 w809 w838 w857 w874 w895 w912 w923]
    tunnel: [w29 w53 w70 w117 w189 w202 w234 w247 w261 w282 w297 w304 w318 w343 w354 w392 w412 w431 w482 w502 w526 w542 w559 w580 w648 w671 w697 w707 w728 w763 w777 w808 w837 w857 w873 w894 w913 w923] -> w17
    tunnel: [w20 w44 _ w115 _ w201 _ w244 w263 w278 _ _ w316 w341 w353 w387 w408 w430 w480 w496 w520 w537 w558 w579 w643 w675 w692 _ w723 w757 _ w804 w833 w856 w869 w889 w907 _] -> w3
    tunnel: [w25 w49 w69 w116 w188 w200 w240 w253 w267 w277 w296 w303 w315 w340 w352 w386 w407 w429 w479 w495 w519 w536 w557 w578 w642 w674 w691 w706 w722 w756 w776 w803 w832 w855 w868 w888 w906 w922] -> w2
    tunnel: w5 -> [w25 w49 w69 w116 w188 w200 w240 w253 w267 w277 w296 w303 w315 w340 w352 w386 w407 w429 w479 w495 w519 w536 w557 w578 _ w674 w691 w706 w722 w756 w776 w803 w832 w855 w868 w888 w906 w922]
    frame "Decay:1-Normalize Decay" {
      # "\"1-Normalize Decay\""
      n4 = Variant To Data(Variant=w32) -> (data=w24:T22, error out=w31:errorcluster)  [unwired: 2 in]
      n5 = call "AlliGator Get Process Plots Indices.vi"("error in (no error)"=w31, "Selected Plot Info"=w24) -> ("error out"=w22:errorcluster, "Selected Plots"=w18:i32[], "Selected Plot Info (dup)"=w23:T22)  [unwired: 7 in]
      n6 = call "XY Graph 1-Normalize Multiple Plots.vi"("error in (no error)"=w22, "Selected Plots"=w18, "Selected Plot Info"=w23) -> ("error out"=w27:errorcluster, "1-Normalize Plot Message"=w20:string, "Last 1-Normalized Plot"=w21:cluster{"t Array":dbl[], "IRF Array":dbl[]}, "Single Plot?"=w19:bool)  [unwired: 5 in]
      n7 = case shown="False" w19 {
        tunnel: [w35 w41] -> w29
        tunnel: w28 -> [w35 w40]
        tunnel: w27 -> [w34 w39]
        tunnel: [w34 w38] -> w26
        tunnel: w21 -> [_ w36]
        frame False {
        }
        frame True {
          n8 = call "AlliGator IV ROI Decay.vi"("Get (F)/ Set (T)"=TRUE, "error in (no error)"=w39, "Decay in"=w36, "AlliGator IV DVR in"=w40) -> ("error out"=w38:errorcluster, "AlliGator IV DVR out"=w41:refnum<data-value>)  [unwired: 4 in, 2 out]
        }
      }
    }
    frame "Decay:[0-1]-Normalize Plot" {
      # "[0-1]-Normalize Plot"
      n9 = Variant To Data(Variant=w56) -> (data=w47:T22, error out=w55:errorcluster)  [unwired: 2 in]
      n10 = call "AlliGator Get Process Plots Indices.vi"("error in (no error)"=w55, "Selected Plot Info"=w47) -> ("error out"=w48:errorcluster, "Selected Plots"=w42:i32[], "Selected Plot Info (dup)"=w46:T22)  [unwired: 7 in]
      n11 = call "XY Graph [0-1]-Normalize Multiple Plots.vi"("error in (no error)"=w48, "Selected Plots"=w42, "Selected Plot Info"=w46) -> ("error out"=w51:errorcluster, "[0-1]-Normalize Plot Message"=w44:string, "Last [0-1]-Normalized Plot"=w45:cluster{"t Array":dbl[], "IRF Array":dbl[]}, "Single Plot?"=w43:bool)  [unwired: 5 in]
      n12 = case shown="True" w43 {
        tunnel: [w59 w65] -> w53
        tunnel: w52 -> [w59 w64]
        tunnel: w51 -> [w58 w63]
        tunnel: [w58 w62] -> w50
        tunnel: w45 -> [_ w61]
        frame False {
        }
        frame True {
          n13 = call "AlliGator IV ROI Decay.vi"("Get (F)/ Set (T)"=TRUE, "error in (no error)"=w63, "Decay in"=w61, "AlliGator IV DVR in"=w64) -> ("error out"=w62:errorcluster, "AlliGator IV DVR out"=w65:refnum<data-value>)  [unwired: 4 in, 2 out]
        }
      }
    }
    frame "Decay:Add Decay Parameter(s) to Plot (Graph)" {
      # "\"Add Decay Parameter(s) to Plot (Graph)\""
      n14 = disable-structure shown="Enabled" {
        disable-tunnel: [w78 w81] -> w68
        disable-tunnel: w67 -> [w77 w81]
        disable-tunnel: [w76 TRUE ("Valid Decay")] -> w66
        frame Disabled {
          n15 = call "AlliGator IV Valid Decay.vi"("Get (F)/ Set (T)"=FALSE, "AlliGator IV DVR in"=w77) -> ("Valid Decay"=w76:bool, "AlliGator IV DVR out"=w78:refnum<data-value>)  [unwired: 7 in, 1 out]
        }
        frame Enabled {
        }
      }
      n16 = case shown="True" w66 {
        tunnel: [_ w104] -> w73
        tunnel: w72 -> [_ w102]
        tunnel: w71 -> [_ w95]
        tunnel: [w82 w85] -> w70
        tunnel: w68 -> [w82 w83]
        frame False {
        }
        frame True {
          w84 = FALSE ("Get (F)/ Set (T)")
          n17 = Unbundle By Name(w95) -> ("Registered Events Ctrl Refnums.Lifetime Graph"=w103:refnum<vi>, "Other AlliGator Ctrl Refnums.Time Step"=w94:refnum<vi>, "Other AlliGator Ctrl Refnums.Use File Timestamp"=w92:refnum<vi>)
          n18 = call "AlliGator IV Single Fit Parameters.vi"("Get (F)/ Set (T)"=w84, "AlliGator IV DVR in"=w83) -> ("error out"=w87:errorcluster, "[Single Decay Fit Parameter]"=w90:dbl[], "AlliGator IV DVR out"=w89:refnum<data-value>)  [unwired: 7 in]
          n19 = property class="Bool (strict)"(reference=w92) -> ("Value"=w91:bool)  [unwired: 1 in, 2 out]
          n20 = call-poly "Variant to Data.vi"("Variant"=w102) -> ("Value"=w100:i32)  [unwired: 8 in]
          n21 = call "AlliGator IV Time Series Timestamps & Current Dataset.vi"("Get (F)/ Set"=w84, "error in (no error)"=w87, "AlliGator IV DVR in"=w89) -> ("Current Dataset"=w88:i32, "[Time-Series Timestamps]"=w86:dbl[], "AlliGator IV DVR out"=w85:refnum<data-value>)  [unwired: 5 in, 1 out]
          n22 = Greater Or Equal To 0?(x=w100) -> (x >= 0?=w101:bool)
          n23 = Select(t=w100, s=w101, f=w88) -> (s? t:f=w99:i32)
          n24 = property class="DigNum (strict)"(reference=w94) -> ("Value"=w93:dbl[unit])  [unwired: 1 in, 2 out]
          n25 = call "AlliGator Get Fit Output Options.vi"("All Parameters?"=FALSE) -> ("Laser Period"=w96:dbl, "Decay Fit Output Options"=w98:T23)  [unwired: 8 in, 1 out]
          n26 = call "AlliGator Get Dataset Series Timestamp & Intensity Correction.vi"("Current Data Set"=w99, "Time Step"=w93, "Use File Timestamp"=w91, "Dataset Series Timestamps"=w86) -> ("Time Stamp (s)"=w108:dbl)  [unwired: 6 in, 1 out]
          n27 = call "Get Decay Fit Parameters.vi"("Laser Period"=w96, "Decay Fit Output Options"=w98, "Decay Fit Parameters"=w90) -> ("Displayed Decay Fits Parameters"=w107:dbl[])  [unwired: 7 in, 1 out]
          n28 = Reverse 1D Array(array=w107) -> (reversed array=w106:dbl[])
          n29 = for {
            tunnel: w103 -> [w114]
            tunnel: w108 -> [w113]
            tunnel: w106 -> [w112] mode=indexing
            tunnel: [w109] -> w105 mode=indexing
            i -> [w111]
            n30 = expression code="-x-1"(w111) -> (w110:i32)
            n31 = call "XY Graph Append Point to Plot.vi"("Plot ID (-1: last)"=w110, "y"=w112, "x"=w113, "XYGraph in"=w114) -> ("error out"=w109:errorcluster)  [unwired: 4 in, 3 out]
          }
          n32 = Merge Errors(w105) -> (w104:errorcluster)
        }
      }
    }
    frame "Decay:Add Decay to Graph" {
      # "\"Add Decay to Graph\""
      n33 = Unbundle By Name(w120) -> ("Other AlliGator Ctrl Refnums.Decay Graph Active"=w121:refnum<vi>)
      n34 = property class="Bool (strict)"(reference=w121) -> ("Value"=w119:bool)  [unwired: 1 in, 2 out]
      n35 = case shown="True" w119 {
        tunnel: w125 -> [w127 w140]
        tunnel: [w127 w139] -> w124
        tunnel: w120 -> [_ w138]
        tunnel: [_ w136] -> w122
        tunnel: w118 -> [w126 w135]
        tunnel: [w126 w130] -> w117
        tunnel: [_ w129] -> w115
        frame False {
        }
        frame True {
          w131 = FALSE ("Get (F)/ Set (T)")
          n36 = Unbundle By Name(w138) -> ("Registered Events Ctrl Refnums.Decay Graph"=w137:refnum<vi>)
          n37 = call "AlliGator IV ROI Decay.vi"("Get (F)/ Set (T)"=w131, "AlliGator IV DVR in"=w135) -> ("error out"=w132:errorcluster, "Valid Decay?"=w128:bool, "Decay out"=w134:cluster{"t Array":dbl[], "IRF Array":dbl[]}, "AlliGator IV DVR out"=w133:refnum<data-value>)  [unwired: 6 in]
          n38 = case shown="True" w128 {
            tunnel: w140 -> [w143 w167]
            tunnel: [w143 w166] -> w139
            tunnel: w137 -> [_ w156]
            tunnel: [w141 w154] -> w136
            tunnel: w134 -> [_ w153]
            tunnel: w133 -> [w142 w152]
            tunnel: w132 -> [w141 w151]
            tunnel: w131 -> [_ w149]
            tunnel: [w142 w147] -> w130
            tunnel: [_ w144] -> w129
            frame False {
            }
            frame True {
              n39 = call "AlliGator IV Current Folder.vi"("Get (F)/ Set (T)"=w149, "error in (no error)"=w151, "AlliGator IV DVR in"=w152) -> ("error out"=w148:errorcluster, "Current Folder"=w150:string, "AlliGator IV DVR out"=w147:refnum<data-value>)  [unwired: 6 in]
              n40 = call "XY Graph Number of Plots.vi"("Error In"=w148, "XYGraph in"=w156) -> ("Error Out"=w155:errorcluster, "# Plots"=w157:i32)  [unwired: 8 in]
              n41 = call "AlliGator New Decay Plot Name.vi"("Current Folder"=w150) -> ("New Decay Name"=w164:string)  [unwired: 8 in]
              n42 = call <userlib>:"MGI Non Repeating Plot Color.vi"("Plot #"=w157) -> ("Color"=w158:u32)
              n43 = call "AlliGator Only Show Last Decay.vi"() -> ("Show Last Decay Only?"=w161:bool)
              n44 = call "XY Graph Add Single Plot with Name.vi"("XYGraph Ref in"=w156, "Plot"=w153, "Plot Name (\"Plot\")"=w164, "error in (no error)"=w155, "Plot Color (Default)"=w158) -> ("XY Graph Caption (or Label)"=w145:string, "Plot Index"=w162:i32, "Plot Name"=w146:string, "error out"=w163:errorcluster)  [unwired: 7 in]
              n45 = call "AlliGator Extract IRF Instead of Decay Flag.vi"() -> ("Extract IRF instead of Decay?"=w165:bool)
              n46 = call "XY Graph Show Plot.vi"("Hide All Other Plots (F)"=w161, "error in (no error)"=w163, "Selected Plot Index"=w162, "XYGraph in"=w156) -> ("error out"=w159:errorcluster, "XYGraph out"=w160:T18)  [unwired: 6 in]
              n47 = case shown="True" w165 {
                tunnel: w160 -> [_ w182]
                tunnel: w167 -> [w174 w180]
                tunnel: [w174 w177] -> w166
                tunnel: w159 -> [w173 w181]
                tunnel: [w172 w175] -> w154
                tunnel: w146 -> [w168 _]
                tunnel: w145 -> [w171 _]
                tunnel: [w169 _] -> w144
                frame False {
                  n48 = Format Into String(format string=" added to %s", initial string=w168, error in=w173, w171) -> (resulting string=w169:string, error out=w172:errorcluster)
                }
                frame True {
                  w183 = T26 {"CtlRef"=refnum, "Coords"={"Horizontal"=0, "Vertical"=0}, "Plot ID"=0}  # IRF Request Event Data
                  n49 = call "XY Graph Get Last Plot ID.vi"("error in (no error)"=w181, "XYGraph in"=w182) -> ("error out"=w178:errorcluster, "Last Plot ID"=w184:i32, "XYGraph out"=w185:refnum<vi>)  [unwired: 7 in]
                  n50 = Bundle By Name(cluster=w183, "CtlRef"=w185, "Plot ID"=w184) -> (w186:T26)
                  n51 = Bundle By Name(cluster=T4 {"AlliGator Q Event"=enum."Decay:Extract IRF", "Data"=variant} ("element"), "Data"=w186) -> (w179:T4)
                  n52 = call-poly "AlliGator Add Action(s) to Stack.vi"("Elements Order in Action Stack (Default: 2 BEFORE 1)"=Alligator_Elements_Order_in_Action_Stack."Enqueue 2 BEFORE 1", "Error In"=w178, "Alligator Atomic Action"=w179, "Alligator Queue Element 1"=w180) -> ("Error Out"=w175:errorcluster, "Alligator Queue Element 1 (+ 2)"=w177:T4[])  [unwired: 6 in]
                }
              }
            }
          }
        }
      }
    }
    frame "Decay:Add Global Fit Parameters to Graph" {
      # "\"Add Global Fit Parameters to Graph\""
      n53 = Unbundle By Name(w194) -> ("Registered Events Ctrl Refnums.Lifetime Graph"=w195:refnum<vi>)
      n54 = call "AlliGator IV Single Fit Parameters.vi"("Get (F)/ Set (T)"=FALSE, "AlliGator IV DVR in"=w193) -> ("error out"=w191:errorcluster, "[Single Decay Fit Parameter]"=w192:dbl[], "AlliGator IV DVR out"=w189:refnum<data-value>)  [unwired: 7 in]
      n55 = call "Plot Global Fit Parameters.vi"("Error In"=w191, "Best Fit Parameters"=w192, "XYGraph in"=w195) -> ("Error Out"=w196:errorcluster)  [unwired: 8 in]
    }
    frame "Decay:Average Selected Plots" {
      # "\"Average Selected Plots\""
      n56 = Variant To Data(Variant=w217) -> (data=w212:refnum<vi>, error out=w209:errorcluster)  [unwired: 2 in]
      n57 = call "Show Animated Busy Icon with Message.vi"("Already active? (F)"=w199, "Message"=w204, "Error In"=w209, "Target VI Refnum"=w203) -> ("Error Out"=w211:errorcluster)  [unwired: 7 in]
      n58 = call "XY Graph Average Selected Plots Event.vi"("Error In"=w211, "XYGraph Ref"=w212) -> ("Error Out"=w210:errorcluster, "Averaged Plot Names"=w215:string[], "Averaged Plot Indices"=w214:i32[], "Graph Label"=w208:string, "Plot Name"=w207:string)  [unwired: 5 in]
      n59 = call "Hide Animated Busy Icon with Message.vi"("Already active? (F)"=w199, "Error In"=w210, "Target VI reference"=w203) -> ("Error Out"=w206:errorcluster)  [unwired: 8 in]
      n60 = Empty Array?(array=w214) -> (empty?=w213:bool)
      n61 = case shown="True" w213 {
        tunnel: w215 -> [w225 _]
        tunnel: w208 -> [w226 _]
        tunnel: w207 -> [w222 _]
        tunnel: w206 -> [w219 w228]
        tunnel: [w221 w228] -> w205
        tunnel: [w218 _] -> w201
        frame False {
          n62 = call "Concatenate String Array.vi"("Max Number of Elements (None: -1)"=5 ("Max Number of Elements (None: 1)"), "Separator (TAB)"=", ", "String Array"=w225) -> ("Formatted String"=w223:string)  [unwired: 8 in]
          n63 = Format Into String(format string="%s in %s: Average of %s", error in=w219, w222, w226, w223) -> (resulting string=w218:string, error out=w221:errorcluster)  [unwired: 1 in]
        }
        frame True {
        }
      }
    }
    frame "Decay:Clear IRF/Reference Plot" {
      w232 = TRUE ("Set (T)/Get")
      # "Clear IRF/Reference Plot"
      n64 = Unbundle By Name(w241) -> ("Other AlliGator Ctrl Refnums.State Indicators"=w237:refnum<vi>)
      n65 = call "AlliGator Get-Set State Indicators.vi"("State Indicators Refnum"=w237, "AlliGator State Indicators List"=AlliGator_State_Indicators_List."Reference/IRF Defined", "ON/OFF"=FALSE, "Set (T)/Get"=w232) -> ("Error Out"=w236:errorcluster)  [unwired: 9 in, 2 out]
      n66 = call "AlliGator IV Reference Decay.vi"("Get (F)/ Set (T)"=w232, "Error In"=w236, "AlliGator IV DVR in"=w235) -> ("Error Out"=w233:errorcluster, "Reference Decay Plot Name"=w230:string, "AlliGator IV DVR out"=w234:refnum<data-value>)  [unwired: 5 in, 1 out]
      n67 = Format Into String(format string="IRF/Reference Plot %s cleared", error in=w233, w230) -> (error out=w231:errorcluster)  [unwired: 1 in, 1 out]
    }
    frame "Decay:Clear Local IRFs" {
      # "\"Decay:Clear Local IRFs\""
      n68 = Unbundle By Name(w254) -> ("Other AlliGator Ctrl Refnums.State Indicators"=w250:refnum<vi>)
      n69 = call "AlliGator Get-Set State Indicators.vi"("State Indicators Refnum"=w250, "AlliGator State Indicators List"=AlliGator_State_Indicators_List."Individual IRFs Defined", "ON/OFF"=FALSE, "Set (T)/Get"=TRUE) -> ("Error Out"=w246:errorcluster)  [unwired: 9 in, 2 out]
      n70 = call "AlliGator Clear Local IRFs.vi"("error in (no error)"=w246, "AlliGator IV DVR in"=w248) -> ("error out"=w245:errorcluster, "Message"=w244:string, "AlliGator IV DVR out"=w247:refnum<data-value>)  [unwired: 7 in]
    }
    frame "Decay:Compute Average Lifetime" {
      # "\"Decay:Compute Average Lifetime\""
      n71 = Variant To Data(Variant=w268) -> (data=w266:T22, error out=w259:errorcluster)  [unwired: 2 in]
      n72 = call "AlliGator Get Reference Decay.vi"("Error In"=w259, "Data Value Reference in"=w262) -> ("Error Out"=w258:errorcluster, "Reference Decay"=w260:cluster{"t Array":dbl[], "I Array":dbl[]}, "Data Value Reference out"=w261:refnum<data-value>)  [unwired: 7 in]
      n73 = call "AlliGator Computer IRF t_0 and Mean Lifetime.vi"("error in"=w258, "Reference Decay"=w260) -> ("error out"=w265:errorcluster, "t_0"=w264:dbl, "<tau>_IRF"=w257:dbl)  [unwired: 7 in]
      n74 = call "AlliGator Get Decay Average Lifetime.vi"("error in (no error)"=w265, "t_0_IRF"=w264, "<tau>_IRF"=w257, "Selected Plot Info"=w266) -> ("Error Out"=w269:errorcluster, "Message"=w263:string)  [unwired: 6 in]
    }
    frame "Decay:Compute Cumulative Function" {
      # "Compute Cumulative Function"
      n75 = Variant To Data(Variant=w286) -> (data=w275:T22, error out=w285:errorcluster)  [unwired: 2 in]
      n76 = call "AlliGator Get Process Plots Indices.vi"("error in (no error)"=w285, "Selected Plot Info"=w275) -> ("error out"=w276:errorcluster, "Selected Plots"=w272:i32[], "Selected Plot Info (dup)"=w274:T22)  [unwired: 7 in]
      n77 = call "XY Graph Cumulative Function of Multiple Plots.vi"("error in (no error)"=w276, "Selected Plots"=w272, "Selected Plot Info"=w274) -> ("error out"=w280:errorcluster, "Cumulative Function Plot Message"=w278:string, "Last Cumulative Function Plot"=w281:cluster{"t Array":dbl[], "IRF Array":dbl[]}, "Single Plot?"=w273:bool)  [unwired: 5 in]
      n78 = case shown="True" w273 {
        tunnel: w283 -> [w289 w295]
        tunnel: [w289 w294] -> w282
        tunnel: w281 -> [_ w293]
        tunnel: w280 -> [w288 w292]
        tunnel: [w288 w291] -> w279
        frame False {
        }
        frame True {
          n79 = call "AlliGator IV ROI Decay.vi"("Get (F)/ Set (T)"=TRUE, "error in (no error)"=w292, "Decay in"=w293, "AlliGator IV DVR in"=w295) -> ("error out"=w291:errorcluster, "AlliGator IV DVR out"=w294:refnum<data-value>)  [unwired: 4 in, 2 out]
        }
      }
    }
    frame "Decay:Create Bounding Cursors Set" {
      # "\"Create Bounding Cursors Set\""
      n80 = Unbundle By Name(w298) -> ("Registered Events Ctrl Refnums.Decay Graph"=w299:refnum<vi>)
      n81 = call "AlliGator Create Cursors for Square Gated IRF Fit.vi"("Decay Graph"=w299) -> ("Error Out"=w300:errorcluster)  [unwired: 9 in, 1 out]
    }
    frame "Decay:Create Head & Tail Bounding Cursors" {
      # "Create Head & Tail Bounding Cursors"
      n82 = Unbundle By Name(w305) -> ("Registered Events Ctrl Refnums.Decay Graph"=w306:refnum<vi>)
      n83 = call "AlliGator Create Head & Tail Bounding Cursors.vi"("Decay Graph"=w306) -> ("Error Out"=w307:errorcluster)  [unwired: 9 in, 1 out]
    }
    frame "Decay:Denoise Plot" {
      # "\"Denoise Plot\""
      n84 = Variant To Data(Variant=w330) -> (data=w313:T22, error out=w329:errorcluster)  [unwired: 2 in]
      n85 = call "AlliGator Get Process Plots Indices.vi"("error in (no error)"=w329, "Selected Plot Info"=w313) -> ("error out"=w314:errorcluster, "Selected Plots"=w311:i32[], "Selected Plot Info (dup)"=w312:T22)  [unwired: 7 in]
      n86 = call "AlliGator Settings Storage.vi"("AlliGator Settings List"=AlliGator_Settings_List."Fluorescence Decay_Advanced Analysis:Wavelet Analysis Options") -> ("Error Out"=w325:errorcluster, "Variant Data out"=w327:variant)  [unwired: 9 in]
      n87 = Variant To Data(error in=w325, Variant=w327) -> (data=w326:T27, error out=w323:errorcluster)  [unwired: 1 in]
      n88 = Merge Errors(w323, w314) -> (w324:errorcluster)
      n89 = call "XY Graph Denoise Multiple Plots.vi"("Wavelet Analysis Options"=w326, "error in (no error)"=w324, "Selected Plots"=w311, "Selected Plot Info"=w312) -> ("error out"=w320:errorcluster, "Denoised Plot Message"=w316:string, "Last Denoised Plot"=w321:cluster{"t Array":dbl[], "IRF Array":dbl[]}, "Single Plot?"=w310:bool)  [unwired: 4 in]
      n90 = case shown="False" w310 {
        tunnel: w321 -> [_ w339]
        tunnel: w320 -> [w332 w338]
        tunnel: [w332 w337] -> w319
        tunnel: [w333 w336] -> w318
        tunnel: w317 -> [w333 w335]
        frame False {
        }
        frame True {
          n91 = call "AlliGator IV ROI Decay.vi"("Get (F)/ Set (T)"=TRUE, "error in (no error)"=w338, "Decay in"=w339, "AlliGator IV DVR in"=w335) -> ("error out"=w337:errorcluster, "AlliGator IV DVR out"=w336:refnum<data-value>)  [unwired: 4 in, 2 out]
        }
      }
    }
    frame "Decay:Export Bounding Cursors Definition to Notebook" {
      # "Export Bounding Cursors Definition to Notebook"
      n92 = Unbundle By Name(w344) -> ("Registered Events Ctrl Refnums.Decay Graph"=w346:refnum<vi>)
      n93 = call "AlliGator Get Square Gated IRF Analysis Cursors.vi"("XYGraph in"=w346) -> ("Error Out"=w349:errorcluster, "Cursor Names Array"=w347:string[], "Cursor Positions Array"=w348:dbl[])  [unwired: 7 in, 1 out]
      n94 = call "AlliGator Square Gated IRF Fit Cursors String.vi"("Error In"=w349, "Cursor Positions Array"=w348, "Cursor Names Array"=w347) -> ("Error Out"=w345:errorcluster, "Message"=w341:string)  [unwired: 7 in]
    }
    frame "Decay:Export Decay to Phasor Graph" {
      # "\"Export Decay to Phasor Graph\""
      n95 = Unbundle By Name(w357) -> ("Phasor Graph Ctrl Refnums.Phasor Graph Active"=w358:refnum<vi>)
      n96 = property class="Bool (strict)"(reference=w358) -> ("Value"=w356:bool)  [unwired: 1 in, 2 out]
      n97 = case shown="True" w356 {
        tunnel: w361 -> [w365 w382]
        tunnel: [w365 w381] -> w360
        tunnel: [_ w378] -> w359
        tunnel: w355 -> [w363 w373]
        tunnel: [w363 w371] -> w354
        tunnel: [_ w370] -> w353
        tunnel: w351 -> [_ w368]
        frame False {
          n98 = One Button Dialog(message="Phasor Graph inactive!") -> ()  [unwired: 1 in, 1 out]
          n99 = call "Play Error Sound.vi"() -> ()  [unwired: 27 in, 1 out]
        }
        frame True {
          w375 = T28 {"Global Rectangle"=[], "Contours"=[{"ID"=enum."External", "Type"=1, "Coordinates"=[]}]}  # Dummy Point
          n100 = Variant To Data(Variant=w368) -> (data=w366:T22, error out=w367:errorcluster)  [unwired: 2 in]
          n101 = call "XY Graph Get Selected Plot.vi"("error in (no error)"=w367, "Selected Plot Info"=w366) -> ("error out"=w372:errorcluster, "Plot Name"=w377:string, "Plot"=w384:T29)  [unwired: 4 in, 3 out]
          n102 = call "AlliGator Get ROI Decay.vi"("error in (no error)"=w372, "Decay"=w384, "ROI Descriptor"=w375, "AlliGator Internal Variables DVR"=w373) -> ("Error Out"=w379:errorcluster, "AlliGator Internal Variables DVR"=w371:refnum<data-value>, "Message"=w369:string)  [unwired: 2 in, 3 out]
          n103 = Format Into String(format string="\n%s's phasor added to Phasor Graph", initial string=w369, error in=w379, w377) -> (resulting string=w370:string, error out=w374:errorcluster)
          n104 = call-poly "AlliGator Add Action(s) to Stack.vi"("Elements Order in Action Stack (Default: 2 BEFORE 1)"=Alligator_Elements_Order_in_Action_Stack."Enqueue 2 BEFORE 1", "Error In"=w374, "Alligator Queue Element 2"=T4[] [{"AlliGator Q Event"=enum."Phasor Graph:Create New Phasor Plot Dialog", "Data"=variant}, {"AlliGator Q Event"=enum."Phasor Graph:Get Phasor Value", "Data"=variant}] ("Alligator Atomic Action"), "Alligator Queue Element 1"=w382) -> ("Error Out"=w378:errorcluster, "Alligator Queue Element 1 (+ 2)"=w381:T4[])  [unwired: 6 in]
        }
      }
    }
    frame "Decay:Extract IRF" {
      # "\"Extract IRF\""
      n105 = Variant To Data(Variant=w400) -> (data=w397:T22, error out=w399:errorcluster)  [unwired: 2 in]
      n106 = call "Show Animated Busy Icon with Message.vi"("Already active? (F)"=w385, "Message"=w395, "Error In"=w399, "Target VI Refnum"=w394) -> ("Error Out"=w396:errorcluster)  [unwired: 7 in]
      n107 = call "Get IRF from Decay v2.vi"("error in (no error)"=w396, "Selected Plot Info"=w397) -> ("Error Out"=w398:errorcluster, "Message"=w387:string, "Extracted IRF"=w389:cluster{"t Array":dbl[], "IRF Array":dbl[]})  [unwired: 7 in]
      n108 = call "Hide Animated Busy Icon with Message.vi"("Already active? (F)"=w385, "Error In"=w398, "Target VI reference"=w394) -> ("Error Out"=w391:errorcluster)  [unwired: 8 in]
      n109 = call "AlliGator IV ROI Decay.vi"("Get (F)/ Set (T)"=TRUE, "error in (no error)"=w391, "Decay in"=w389, "AlliGator IV DVR in"=w393) -> ("error out"=w390:errorcluster, "AlliGator IV DVR out"=w392:refnum<data-value>)  [unwired: 4 in, 2 out]
    }
    frame "Decay:Extrapolate Decay" {
      # "\"Extrapolate Decay\""
      n110 = Variant To Data(Variant=w416) -> (data=w405:T22, error out=w415:errorcluster)  [unwired: 2 in]
      n111 = call "AlliGator Get Process Plots Indices.vi"("error in (no error)"=w415, "Selected Plot Info"=w405) -> ("error out"=w406:errorcluster, "Selected Plots"=w403:i32[], "Selected Plot Info (dup)"=w404:T22)  [unwired: 7 in]
      n112 = call "AlliGator Extrapolate Multiple Plots.vi"("error in (no error)"=w406, "Selected Plots"=w403, "Selected Plot Info"=w404) -> ("error out"=w410:errorcluster, "Extrapolated Decay Message"=w408:string, "Last Extrapolated Decay"=w411:cluster{"t Array":dbl[], "IRF Array":dbl[]}, "Single Plot?"=w402:bool)  [unwired: 5 in]
      n113 = case shown="True" w402 {
        tunnel: w413 -> [w419 w425]
        tunnel: [w419 w424] -> w412
        tunnel: w411 -> [_ w423]
        tunnel: w410 -> [w418 w422]
        tunnel: [w418 w421] -> w409
        frame False {
        }
        frame True {
          n114 = call "AlliGator IV ROI Decay.vi"("Get (F)/ Set (T)"=TRUE, "error in (no error)"=w422, "Decay in"=w423, "AlliGator IV DVR in"=w425) -> ("error out"=w421:errorcluster, "AlliGator IV DVR out"=w424:refnum<data-value>)  [unwired: 4 in, 2 out]
        }
      }
    }
    frame "Decay:Fit Decay" {
      # "\"Fit Decay\""
      n115 = disable-structure shown="Enabled" {
        disable-tunnel: [w441 w443] -> w428
        disable-tunnel: w427 -> [w440 w443]
        disable-tunnel: [w438 TRUE ("Valid Decay")] -> w426
        frame Disabled {
          n116 = call "AlliGator IV Valid Decay.vi"("Get (F)/ Set (T)"=FALSE, "AlliGator IV DVR in"=w440) -> ("Valid Decay"=w438:bool, "AlliGator IV DVR out"=w441:refnum<data-value>)  [unwired: 7 in, 1 out]
        }
        frame Enabled {
        }
      }
      n117 = case shown="True" w426 {
        tunnel: w436 -> [_ w475]
        tunnel: [_ w474] -> w435
        tunnel: w434 -> [_ w473]
        tunnel: w433 -> [_ w472]
        tunnel: w432 -> [_ w471]
        tunnel: [w444 w465] -> w431
        tunnel: [_ w464] -> w430
        tunnel: w428 -> [w444 w463]
        frame False {
        }
        frame True {
          w458 = "Abort Fit" ("Abort Button Name (Abort)")
          n118 = call "AlliGator Check Decay Reference.vi"("AlliGator Internal Variables DVR"=w463) -> ("Error Out"=w469:errorcluster, "Reference Decay"=w446:cluster{"t Array":dbl[], "I Array":dbl[]}, "AlliGator Internal Variables DVR"=w470:refnum<data-value>)  [unwired: 3 in, 5 out]
          n119 = call "AlliGator IV ROI Decay.vi"("Get (F)/ Set (T)"=FALSE, "error in (no error)"=w469, "AlliGator IV DVR in"=w470) -> ("error out"=w468:errorcluster, "Decay out"=w467:cluster{"t Array":dbl[], "IRF Array":dbl[]}, "AlliGator IV DVR out"=w466:refnum<data-value>)  [unwired: 5 in, 1 out]
          n120 = Variant To Data(error in=w468, type=T17 {"Multiplot XY Graph"=refnum, "Mouse Coordinates"={"Horizontal"=0, "Vertical"=0}, "Plot Index"=-1, "Flag"=FALSE} ("Selected Plot Info + Flag"), Variant=w475) -> (data=w457:T17, error out=w462:errorcluster)
          n121 = call "Show Animated Busy Icon with Message and Abort Button.vi"("Already active? (F)"=w473, "Message"=w472, "Target VI reference"=w471, "Error In"=w462, "Abort Button Name (Abort)"=w458) -> ("Error Out"=w451:errorcluster)  [unwired: 14 in]
          n122 = call "AlliGator Get Fit Options & Parameters.vi"("error in (no error)"=w451, "Reset Fit Options & Parameters"=TRUE) -> ("error out"=w450:errorcluster, "Use Legacy Fitting Approach"=w449:bool, "Decay Fit Options & Parameters"=w448:T30)  [unwired: 7 in]
          n123 = call "AlliGator Fit Decay.vi"("Selected Plot Info + Flag"=w457, "Decay Fit Options & Parameters"=w448, "Current Decay"=w467, "Reference Decay"=w446, "error in (no error)"=w450, "Use Legacy Fitting Approach"=w449) -> ("Best Fit Parameters (All)"=w461:dbl[], "R^2"=w460:dbl, "Reduced Chi^2"=w459:dbl, "Fit Output Message"=w464:string, "Error Out"=w453:errorcluster)  [unwired: 1 in, 4 out]
          n124 = Build Array (concatenate)(w461, w460, w459) -> (w455:dbl[])
          n125 = call "AlliGator IV Single Fit Parameters.vi"("Get (F)/ Set (T)"=TRUE, "error in (no error)"=w453, "[Single Decay Fit Parameter]"=w455, "AlliGator IV DVR in"=w466) -> ("error out"=w452:errorcluster, "AlliGator IV DVR out"=w465:refnum<data-value>)  [unwired: 5 in, 1 out]
          n126 = call "Hide Animated Busy Icon with Message and Abort Button.vi"("Already active? (F)"=w473, "Target VI reference"=w471, "Error In"=w452, "Abort Button Name (Abort)"=w458) -> ("Error Out"=w474:errorcluster)  [unwired: 15 in]
        }
      }
    }
    frame "Decay:Fit IRF to Logistic Square Gate" {
      # "Fit IRF to Logistic Square Gate"
      n127 = Variant To Data(Variant=w478) -> (data=w477:T22, error out=w492:errorcluster)  [unwired: 2 in]
      n128 = call "Show Animated Busy Icon with Message.vi"("Already active? (F)"=w476, "Message"=w485, "Error In"=w492, "Target VI Refnum"=w486) -> ("Error Out"=w490:errorcluster)  [unwired: 7 in]
      n129 = call "AlliGator Fit to Logistic Square Gated IRF.vi"("error in (no error)"=w490, "Selected Plot Info"=w477) -> ("Error Out"=w491:errorcluster, "Message"=w480:string, "Fitted IRF"=w488:cluster{"t Array":dbl[], "IRF Array":dbl[]})  [unwired: 7 in]
      n130 = call "Hide Animated Busy Icon with Message.vi"("Already active? (F)"=w476, "Error In"=w491, "Target VI reference"=w486) -> ("Error Out"=w489:errorcluster)  [unwired: 8 in]
      n131 = call "AlliGator IV ROI Decay.vi"("Get (F)/ Set (T)"=TRUE, "error in (no error)"=w489, "Decay in"=w488, "AlliGator IV DVR in"=w483) -> ("error out"=w481:errorcluster, "AlliGator IV DVR out"=w482:refnum<data-value>)  [unwired: 4 in, 2 out]
    }
    frame "Decay:Fit IRF to Square Gate" {
      # "\"Fit IRF to Square Gate\""
      n132 = Variant To Data(Variant=w515) -> (data=w494:T22, error out=w511:errorcluster)  [unwired: 2 in]
      n133 = call "AlliGator Settings Storage.vi"("AlliGator Settings List"=AlliGator_Settings_List."Fluorescence Decay_Advanced Analysis:Square Pulse Options", "Error In"=w511) -> ("Error Out"=w509:errorcluster, "Variant Data out"=w510:variant)  [unwired: 8 in]
      n134 = call "Show Animated Busy Icon with Message.vi"("Already active? (F)"=w493, "Message"=w503, "Error In"=w511, "Target VI Refnum"=w504) -> ("Error Out"=w513:errorcluster)  [unwired: 7 in]
      n135 = Variant To Data(error in=w509, type=T20 {"Method"=enum."Mode", "# Bins"=100, "Threshold %"=10.0, "Center on Midpoint"=TRUE, "Smoothen Plot"=FALSE} ("Square Pulse Options"), Variant=w510) -> (data=w505:T20, error out=w506:errorcluster)
      n136 = Merge Errors(w513, w506) -> (w507:errorcluster)
      n137 = call "Fit to Square Pulse.vi"("Square Pulse Options"=w505, "error in (no error)"=w507, "Selected Plot Info"=w494) -> ("Error Out"=w514:errorcluster, "Fitted Plot Message"=w496:string, "Fitted Plot"=w500:T40)  [unwired: 6 in]
      n138 = call "Hide Animated Busy Icon with Message.vi"("Already active? (F)"=w493, "Error In"=w514, "Target VI reference"=w504) -> ("Error Out"=w499:errorcluster)  [unwired: 8 in]
      n139 = call "AlliGator IV ROI Decay.vi"("Get (F)/ Set (T)"=TRUE, "error in (no error)"=w499, "Decay in"=w500, "AlliGator IV DVR in"=w501) -> ("error out"=w498:errorcluster, "AlliGator IV DVR out"=w502:refnum<data-value>)  [unwired: 4 in, 2 out]
    }
    frame "Decay:Fit IRF to Tilted Logistic Square Gate" {
      # "\"Fit IRF to Tilted Logistic Square Gate\""
      n140 = Variant To Data(Variant=w532) -> (data=w518:T22, error out=w531:errorcluster)  [unwired: 2 in]
      n141 = call "Show Animated Busy Icon with Message.vi"("Already active? (F)"=w517, "Message"=w527, "Error In"=w531, "Target VI Refnum"=w528) -> ("Error Out"=w529:errorcluster)  [unwired: 7 in]
      n142 = call "AlliGator Fit to Tilted Logistic Square Gated IRF.vi"("error in (no error)"=w529, "Selected Plot Info"=w518) -> ("Error Out"=w530:errorcluster, "Message"=w520:string, "Fitted IRF"=w522:cluster{"t Array":dbl[], "IRF Array":dbl[]})  [unwired: 7 in]
      n143 = call "Hide Animated Busy Icon with Message.vi"("Already active? (F)"=w517, "Error In"=w530, "Target VI reference"=w528) -> ("Error Out"=w524:errorcluster)  [unwired: 8 in]
      n144 = call "AlliGator IV ROI Decay.vi"("Get (F)/ Set (T)"=TRUE, "error in (no error)"=w524, "Decay in"=w522, "AlliGator IV DVR in"=w525) -> ("error out"=w523:errorcluster, "AlliGator IV DVR out"=w526:refnum<data-value>)  [unwired: 4 in, 2 out]
    }
    frame "Decay:Fit to Model IRF" {
      # "\"Fit to Model IRF\""
      n145 = Variant To Data(Variant=w549) -> (data=w535:T22, error out=w548:errorcluster)  [unwired: 2 in]
      n146 = call "Show Animated Busy Icon with Message.vi"("Already active? (F)"=w534, "Message"=w544, "Error In"=w548, "Target VI Refnum"=w545) -> ("Error Out"=w546:errorcluster)  [unwired: 7 in]
      n147 = call "AlliGator Fit to Model IRF.vi"("error in (no error)"=w546, "Selected Plot Info"=w535) -> ("Error Out"=w547:errorcluster, "Message"=w537:string, "Fitted IRF"=w541:cluster{"t Array":dbl[], "IRF Array":dbl[]})  [unwired: 7 in]
      n148 = call "Hide Animated Busy Icon with Message.vi"("Already active? (F)"=w534, "Error In"=w547, "Target VI reference"=w545) -> ("Error Out"=w540:errorcluster)  [unwired: 8 in]
      n149 = call "AlliGator IV ROI Decay.vi"("Get (F)/ Set (T)"=TRUE, "error in (no error)"=w540, "Decay in"=w541, "AlliGator IV DVR in"=w543) -> ("error out"=w539:errorcluster, "AlliGator IV DVR out"=w542:refnum<data-value>)  [unwired: 4 in, 2 out]
    }
    frame "Decay:Fold Decay" {
      # "\"Fold Decay\""
      n150 = Variant To Data(Variant=w568) -> (data=w554:T22, error out=w556:errorcluster)  [unwired: 2 in]
      n151 = call "AlliGator Get Process Plots Indices.vi"("error in (no error)"=w556, "Selected Plot Info"=w554) -> ("error out"=w555:errorcluster, "Selected Plots"=w552:i32[], "Selected Plot Info (dup)"=w553:T22)  [unwired: 7 in]
      n152 = call "AlliGator Settings Storage.vi"("AlliGator Settings List"=AlliGator_Settings_List."Fluorescence Decay_Decay Pre-Processing:# Folds") -> ("Variant Data out"=w565:variant)  [unwired: 9 in, 1 out]
      n153 = call-poly "Variant to Data.vi"("Variant"=w565) -> ("Value"=w564:u32)  [unwired: 8 in]
      n154 = call "XY Graph Fold Multiple Plots.vi"("error in (no error)"=w555, "# Folds (1)"=w564, "Selected Plots"=w552, "Selected Plot Info"=w553) -> ("error out"=w562:errorcluster, "Folded Plot Message"=w558:string, "Last Folded Plot"=w560:cluster{"t Array":dbl[], "IRF Array":dbl[]}, "Single Plot?"=w551:bool)  [unwired: 4 in]
      n155 = case shown="False" w551 {
        tunnel: w563 -> [w571 w577]
        tunnel: w562 -> [w570 w576]
        tunnel: [w570 w575] -> w561
        tunnel: w560 -> [_ w574]
        tunnel: [w571 w573] -> w559
        frame False {
        }
        frame True {
          n156 = call "AlliGator IV ROI Decay.vi"("Get (F)/ Set (T)"=TRUE, "error in (no error)"=w576, "Decay in"=w574, "AlliGator IV DVR in"=w577) -> ("error out"=w575:errorcluster, "AlliGator IV DVR out"=w573:refnum<data-value>)  [unwired: 4 in, 2 out]
        }
      }
    }
    frame "Decay:Global Fit of Selected Decays" {
      # "\"Global Fit of Selected Decays\""
      n157 = disable-structure shown="Enabled" {
        disable-tunnel: [w605 _] -> w588
        disable-tunnel: w587 -> [w604 w639]
        disable-tunnel: [w603 w639] -> w586
        disable-tunnel: w585 -> [w602 _]
        disable-tunnel: w584 -> [w597 _]
        disable-tunnel: w583 -> [w596 _]
        disable-tunnel: w582 -> [w594 _]
        disable-tunnel: w581 -> [w593 w640]
        disable-tunnel: [w591 w640] -> w580
        disable-tunnel: [w589 _] -> w579
        frame Disabled {
          n158 = Unbundle By Name(w597) -> ("Registered Events Ctrl Refnums.Decay Graph"=w601:refnum<vi>, "Other AlliGator Ctrl Refnums.Abort Fit"=w595:refnum<vi>)
          n159 = call "AlliGator Check Decay Reference.vi"("AlliGator Internal Variables DVR"=w593) -> ("Error Out"=w590:errorcluster, "Valid Reference?"=w600:bool, "Reference Decay"=w598:cluster{"t Array":dbl[], "I Array":dbl[]}, "AlliGator Internal Variables DVR"=w592:refnum<data-value>, "Message"=w599:string)  [unwired: 3 in, 3 out]
          n160 = case shown="True" w600 {
            tunnel: [w608 w637] -> w589
            tunnel: [w606 w612] -> w605
            tunnel: w604 -> [w609 w628]
            tunnel: [w609 w629] -> w603
            tunnel: w602 -> [_ w610]
            tunnel: w601 -> [_ w623]
            tunnel: w599 -> [w608 _]
            tunnel: w598 -> [_ w622]
            tunnel: w596 -> [_ w621]
            tunnel: w595 -> [_ w620]
            tunnel: w594 -> [_ w619]
            tunnel: [w607 w615] -> w591
            tunnel: w592 -> [w607 w618]
            tunnel: w590 -> [w606 _]
            frame False {
            }
            frame True {
              n161 = call "Show Animated Busy Icon with Message.vi"("Already active? (F)"=w610, "Message"=w619, "Target VI Refnum"=w621) -> ("Error Out"=w635:errorcluster)  [unwired: 8 in]
              n162 = call "Global Fit Decays.vi"("IRF"=w622, "error in (no error)"=w635, "Abort Fit"=w620, "Decay Graph"=w623) -> ("Error Out"=w617:errorcluster, "Reduced Chi^2"=w624:dbl, "R^2"=w625:dbl, "Best Fit Parameters"=w636:dbl[], "Fit Output Message"=w637:string, "Aborted?"=w634:bool)  [unwired: 2 in]
              n163 = Build Array (concatenate)(w636, w625, w624) -> (w616:dbl[])
              n164 = call "AlliGator IV Single Fit Parameters.vi"("Get (F)/ Set (T)"=TRUE, "error in (no error)"=w617, "[Single Decay Fit Parameter]"=w616, "AlliGator IV DVR in"=w618) -> ("error out"=w614:errorcluster, "AlliGator IV DVR out"=w615:refnum<data-value>)  [unwired: 5 in, 1 out]
              n165 = Select(t="Fit Aborted!" ("Fit Output Message"), s=w634, f="") -> (s? t:f=w631:string)
              n166 = call "Play Error Sound.vi"("Error In"=w614) -> ("Error Out"=w630:errorcluster)  [unwired: 26 in]
              n167 = call "Hide Animated Busy Icon with Message.vi"("Already active? (F)"=w610, "Message"=w631, "Error In"=w630, "Target VI reference"=w621) -> ("Error Out"=w613:errorcluster)  [unwired: 7 in]
              n168 = flat-sequence {
                tunnel: w612 -> [_]
                frame #0 {
                  n169 = global write "Abort Fit Global.vi" "Abort Fit"(FALSE ("Visible")) -> ()
                }
              }
              n170 = call-poly "AlliGator Add Action(s) to Stack.vi"("Elements Order in Action Stack (Default: 2 BEFORE 1)"=Alligator_Elements_Order_in_Action_Stack."Enqueue 2 BEFORE 1", "Error In"=w613, "Alligator Atomic Action"=T4 {"AlliGator Q Event"=enum."Decay:Post Global Fit Script", "Data"=variant}, "Alligator Queue Element 1"=w628) -> ("Error Out"=w612:errorcluster, "Alligator Queue Element 1 (+ 2)"=w629:T4[])  [unwired: 6 in]
            }
          }
        }
        frame Enabled {
        }
      }
    }
    frame "Decay:Optimal IRF Extraction" {
      # "\"Optimal IRF Extraction\""
      n171 = Variant To Data(Variant=w656) -> (data=w652:T22, error out=w655:errorcluster)  [unwired: 2 in]
      n172 = call "Show Animated Busy Icon with Message.vi"("Already active? (F)"=w641, "Message"=w651, "Error In"=w655, "Target VI Refnum"=w650) -> ("Error Out"=w653:errorcluster)  [unwired: 7 in]
      n173 = call "AlliGator Get Optimal IRF from Decay v2.vi"("error in (no error)"=w653, "Selected Plot Info"=w652) -> ("Error Out"=w654:errorcluster, "Message Style"=w642:T2, "Message"=w643:string, "Extracted IRF"=w645:cluster{"t Array":dbl[], "IRF Array":dbl[]})  [unwired: 6 in]
      n174 = call "Hide Animated Busy Icon with Message.vi"("Already active? (F)"=w641, "Error In"=w654, "Target VI reference"=w650) -> ("Error Out"=w647:errorcluster)  [unwired: 8 in]
      n175 = call "AlliGator IV ROI Decay.vi"("Get (F)/ Set (T)"=TRUE, "error in (no error)"=w647, "Decay in"=w645, "AlliGator IV DVR in"=w649) -> ("error out"=w646:errorcluster, "AlliGator IV DVR out"=w648:refnum<data-value>)  [unwired: 4 in, 2 out]
    }
    frame "Decay:Plot Convolution" {
      # "\"Decay:Plot Convolution\""
      n176 = Variant To Data(type=T22 {"Multiplot XY Graph"=refnum, "Mouse Coordinates"={"Horizontal"=0, "Vertical"=0}, "Plot Index"=-1} ("Selected Plot Info"), Variant=w680) -> (data=w670:T22, error out=w666:errorcluster)  [unwired: 1 in]
      n177 = call "AlliGator IV Reference Decay.vi"("Get (F)/ Set (T)"=FALSE, "Error In"=w666, "AlliGator IV DVR in"=w673) -> ("Error Out"=w667:errorcluster, "Reference Decay"=w668:cluster{"t Array":dbl[], "I Array":dbl[]}, "AlliGator IV DVR out"=w671:refnum<data-value>)  [unwired: 5 in, 1 out]
      n178 = call "AlliGator Get Selected Plots and Reference Decay.vi"("error in (no error)"=w667, "Reference Decay"=w668, "Selected Plot Info"=w670) -> ("error out"=w663:errorcluster, "Valid Reference Decay?"=w664:bool, "Selected Plots"=w661:i32[], "XYGraph"=w665:T18, "Reference Decay"=w662:cluster{"t Array":dbl[], "Value Array":dbl[]})  [unwired: 4 in]
      n179 = for {
        tunnel: [w690] -> w660 mode=indexing if=w682
        tunnel: w665 -> [w688]
        tunnel: w664 -> [w687]
        tunnel: w662 -> [w685]
        tunnel: w661 -> [w684] mode=indexing
        tunnel: w663 -> [w686]
        n180 = call "XY Graph Compute Convolution Product Event.vi"("Reference Decay"=w685, "Error In"=w686, "Valid Reference Decay?"=w687, "Plot at Coordinates"=w684, "Multiplot XY Graph"=w688) -> ("Error Out"=w689:errorcluster, "Message"=w690:string)  [unwired: 4 in, 1 out]
        n181 = Unbundle By Name(w689) -> ("status"=w683:bool)
        n182 = Not(x=w683) -> (.not. x?=w682:bool)
      }
      n183 = call <vilib>:"1D String Array to Delimited String.vi"("delimiter"="\n", "string array"=w660) -> ("delimited string"=w658:string)  [unwired: 9 in]
      n184 = Format Into String(format string="%s: %s", w678, w658) -> (resulting string=w675:string, error out=w677:errorcluster)  [unwired: 2 in]
    }
    frame "Decay:Plot Decay Shifts" {
      # "\"Plot Decay Shifts\""
      n185 = Unbundle By Name(w698) -> ("Registered Events Ctrl Refnums.Lifetime Graph"=w699:refnum<vi>)
      n186 = call "AlliGator IV Decay Shift Plot.vi"("Get (F)/ Set (T)"=FALSE, "AlliGator IV DVR in"=w696) -> ("error out"=w694:errorcluster, "Decay Shift Plot out"=w695:cluster{"t Array":dbl[], "IRF Array":dbl[]}, "AlliGator IV DVR out"=w697:refnum<data-value>)  [unwired: 7 in]
      n187 = call "XY Graph Add Single Plot with Name.vi"("XYGraph Ref in"=w699, "Plot"=w695, "Plot Name (\"Plot\")"="Decay Shifts" ("Plot Name (\"Plot\")"), "error in (no error)"=w694) -> ("Plot Name"=w703:string, "error out"=w701:errorcluster)  [unwired: 8 in, 2 out]
      n188 = Concatenate Strings(w703, " added to Lifetime & Other Parameters Graph" ("format string")) -> (w692:string)
    }
    frame "Decay:Post Global Fit Script" {
      # "\"Post Global Fit Script\""
      n189 = Unbundle By Name(w714) -> ("Registered Events Ctrl Refnums.Lifetime Graph"=w715:refnum<vi>)
      n190 = call "Post Global Fit Script.vi"("XYGraph in"=w715) -> ("Error Out"=w710:errorcluster, "Q Elements out"=w711:T4[])  [unwired: 9 in]
      n191 = call-poly "AlliGator Add Action(s) to Stack.vi"("Elements Order in Action Stack (Default: 2 BEFORE 1)"=Alligator_Elements_Order_in_Action_Stack."Enqueue 2 BEFORE 1", "Error In"=w710, "Alligator Queue Element 2"=w711, "Alligator Queue Element 1"=w713) -> ("Error Out"=w709:errorcluster, "Alligator Queue Element 1 (+ 2)"=w712:T4[])  [unwired: 6 in]
    }
    frame "Decay:Rebin Plot" {
      # "\"Decay:Rebin Plot\""
      n192 = Variant To Data(Variant=w731) -> (data=w720:T22, error out=w730:errorcluster)  [unwired: 2 in]
      n193 = call "AlliGator Get Process Plots Indices.vi"("error in (no error)"=w730, "Selected Plot Info"=w720) -> ("error out"=w721:errorcluster, "Selected Plots"=w717:i32[], "Selected Plot Info (dup)"=w719:T22)  [unwired: 7 in]
      n194 = call "XY Graph Rebin Multiple Plots.vi"("error in (no error)"=w721, "Selected Plots"=w717, "Selected Plot Info"=w719) -> ("error out"=w725:errorcluster, "Rebinned Plot Message"=w723:string, "Last Rebinned Plot"=w726:cluster{"t Array":dbl[], "IRF Array":dbl[]}, "Single Plot?"=w718:bool)  [unwired: 5 in]
      n195 = case shown="True" w718 {
        tunnel: [w734 w740] -> w728
        tunnel: w727 -> [w734 w739]
        tunnel: w726 -> [_ w738]
        tunnel: w725 -> [w733 w737]
        tunnel: [w733 w736] -> w724
        frame False {
        }
        frame True {
          n196 = call "AlliGator IV ROI Decay.vi"("Get (F)/ Set (T)"=TRUE, "error in (no error)"=w737, "Decay in"=w738, "AlliGator IV DVR in"=w739) -> ("error out"=w736:errorcluster, "AlliGator IV DVR out"=w740:refnum<data-value>)  [unwired: 4 in, 2 out]
        }
      }
    }
    frame "Decay:Shift Decay" {
      # "\"Shift Decay\""
      n197 = Variant To Data(Variant=w766) -> (data=w752:T22, error out=w754:errorcluster)  [unwired: 2 in]
      n198 = call "AlliGator IV Reference Decay.vi"("Get (F)/ Set (T)"=FALSE, "AlliGator IV DVR in"=w761) -> ("Error Out"=w749:errorcluster, "Reference Decay"=w760:cluster{"t Array":dbl[], "I Array":dbl[]}, "AlliGator IV DVR out"=w759:refnum<data-value>)  [unwired: 6 in, 1 out]
      n199 = call "AlliGator Settings Storage.vi"("Get(F)/Set"=FALSE, "AlliGator Settings List"=AlliGator_Settings_List."Fluorescence Decay_Decay Pre-Processing:Decay Shift Parameters") -> ("Error Out"=w747:errorcluster, "Variant Data out"=w748:variant)  [unwired: 8 in]
      n200 = call "AlliGator Get Process Plots Indices.vi"("error in (no error)"=w754, "Selected Plot Info"=w752) -> ("error out"=w753:errorcluster, "Selected Plots"=w742:i32[], "Selected Plot Info (dup)"=w751:T22)  [unwired: 7 in]
      n201 = Variant To Data(error in=w747, Variant=w748) -> (data=w743:T41, error out=w744:errorcluster)  [unwired: 1 in]
      n202 = Merge Errors(w753, w749, w744) -> (w750:errorcluster)
      n203 = call "XY Graph Shift Multiple Plots.vi"("Plot Shift Parameters"=w743, "Reference Decay"=w760, "error in (no error)"=w750, "Selected Plots"=w742, "Selected Plot Info"=w751) -> ("error out"=w755:errorcluster, "Shifted Plot Message"=w757:string, "Last Shifted Plot"=w764:cluster{"t Array":dbl[], "IRF Array":dbl[]}, "Single Plot?"=w741:bool)  [unwired: 3 in]
      n204 = case shown="True" w741 {
        tunnel: w764 -> [_ w775]
        tunnel: [w769 w774] -> w763
        tunnel: [w768 w773] -> w762
        tunnel: w759 -> [w769 w771]
        tunnel: w755 -> [w768 w770]
        frame False {
        }
        frame True {
          n205 = call "AlliGator IV ROI Decay.vi"("Get (F)/ Set (T)"=TRUE, "error in (no error)"=w770, "Decay in"=w775, "AlliGator IV DVR in"=w771) -> ("error out"=w773:errorcluster, "AlliGator IV DVR out"=w774:refnum<data-value>)  [unwired: 4 in, 2 out]
        }
      }
    }
    frame "Decay:Show Reference Decay/IRF" {
      # "\"Show Reference Decay/IRF\""
      n206 = Unbundle By Name(w780) -> ("Registered Events Ctrl Refnums.Decay Graph"=w784:refnum<vi>)
      n207 = call "AlliGator Check Decay Reference.vi"("AlliGator Internal Variables DVR"=w779) -> ("Error Out"=w778:errorcluster, "Valid Reference?"=w781:bool, "Reference Decay"=w783:cluster{"t Array":dbl[], "I Array":dbl[]}, "AlliGator Internal Variables DVR"=w777:refnum<data-value>, "Reference Decay Plot Name"=w782:string)  [unwired: 3 in, 3 out]
      n208 = case shown="False" w781 {
        tunnel: w782 -> [_ w793]
        tunnel: w783 -> [_ w794]
        tunnel: w784 -> [_ w795]
        tunnel: [w788 w791] -> w785
        tunnel: w778 -> [w788 w790]
        frame False {
          n209 = One Button Dialog(message="No Valid Reference Decay/IRF !") -> ()  [unwired: 1 in, 1 out]
          n210 = call "Play Error Sound.vi"() -> ()  [unwired: 27 in, 1 out]
        }
        frame True {
          w792 = T43 6 items=["Point (.)", "Stepwise Right (--.)", "Line + Point (\\. /)", "Stepwise Left (.--)", "Stepwise Centered (-.-)", "Stepwise Vertical (|.|)", "Line (-)", "Use Previous Plot's Style"] ("Plot Interpolation (Previous Plot's Style)")
          n211 = call-poly "XY Graph Add Plot(s) with Name(s).vi"("XYGraph Ref in"=w795, "Plot Interpolation (Previous Plot's Style)"=w792, "Plot"=w794, "Plot Name (\"Plot\")"=w793, "error in (no error)"=w790) -> ("error out"=w791:errorcluster)  [unwired: 7 in, 3 out]
        }
      }
    }
    frame "Decay:Smoothen Plot Tail" {
      # "\"Smoothen Plot\""
      n212 = Variant To Data(Variant=w815) -> (data=w800:T22, error out=w814:errorcluster)  [unwired: 2 in]
      n213 = call "AlliGator Settings Storage.vi"("AlliGator Settings List"=AlliGator_Settings_List."Fluorescence Decay_Decay Pre-Processing:Smoothing Parameter") -> ("Variant Data out"=w812:variant)  [unwired: 9 in, 1 out]
      n214 = call-poly "Variant to Data.vi"("Variant"=w812) -> ("Value"=w811:dbl)  [unwired: 8 in]
      n215 = call "AlliGator Get Process Plots Indices.vi"("error in (no error)"=w814, "Selected Plot Info"=w800) -> ("error out"=w801:errorcluster, "Selected Plots"=w798:i32[], "Selected Plot Info (dup)"=w799:T22)  [unwired: 7 in]
      n216 = expression code="1-10**(-x)"(w811) -> (w802:dbl)
      n217 = call "XY Graph Smoothen Multiple Plots (Cubic Spline).vi"("balance parameter (-1: auto)"=w802, "error in (no error)"=w801, "Tail only (F)"=TRUE, "Selected Plots"=w798, "Selected Plot Info"=w799) -> ("error out"=w805:errorcluster, "Smoothened Plot Message"=w804:string, "Last Smoothened Plot"=w807:cluster{"t Array":dbl[], "IRF Array":dbl[]}, "Single Plot?"=w796:bool)  [unwired: 3 in]
      n218 = case shown="True" w796 {
        tunnel: w809 -> [w818 w824]
        tunnel: [w818 w823] -> w808
        tunnel: w807 -> [_ w822]
        tunnel: [w817 w821] -> w806
        tunnel: w805 -> [w817 w820]
        frame False {
        }
        frame True {
          n219 = call "AlliGator IV ROI Decay.vi"("Get (F)/ Set (T)"=TRUE, "error in (no error)"=w820, "Decay in"=w822, "AlliGator IV DVR in"=w824) -> ("error out"=w821:errorcluster, "AlliGator IV DVR out"=w823:refnum<data-value>)  [unwired: 4 in, 2 out]
        }
      }
    }
    frame "Decay:Smoothen Plot" {
      # "\"Smoothen Plot\""
      n220 = Variant To Data(Variant=w844) -> (data=w829:T22, error out=w843:errorcluster)  [unwired: 2 in]
      n221 = call "AlliGator Settings Storage.vi"("AlliGator Settings List"=AlliGator_Settings_List."Fluorescence Decay_Decay Pre-Processing:Smoothing Parameter") -> ("Variant Data out"=w841:variant)  [unwired: 9 in, 1 out]
      n222 = call-poly "Variant to Data.vi"("Variant"=w841) -> ("Value"=w840:dbl)  [unwired: 8 in]
      n223 = call "AlliGator Get Process Plots Indices.vi"("error in (no error)"=w843, "Selected Plot Info"=w829) -> ("error out"=w830:errorcluster, "Selected Plots"=w827:i32[], "Selected Plot Info (dup)"=w828:T22)  [unwired: 7 in]
      n224 = expression code="1-10**(-x)"(w840) -> (w831:dbl)
      n225 = call "XY Graph Smoothen Multiple Plots (Cubic Spline).vi"("balance parameter (-1: auto)"=w831, "error in (no error)"=w830, "Tail only (F)"=FALSE, "Selected Plots"=w827, "Selected Plot Info"=w828) -> ("error out"=w834:errorcluster, "Smoothened Plot Message"=w833:string, "Last Smoothened Plot"=w836:cluster{"t Array":dbl[], "IRF Array":dbl[]}, "Single Plot?"=w825:bool)  [unwired: 3 in]
      n226 = case shown="True" w825 {
        tunnel: w838 -> [w847 w853]
        tunnel: [w847 w852] -> w837
        tunnel: w836 -> [_ w851]
        tunnel: [w846 w850] -> w835
        tunnel: w834 -> [w846 w849]
        frame False {
        }
        frame True {
          n227 = call "AlliGator IV ROI Decay.vi"("Get (F)/ Set (T)"=TRUE, "error in (no error)"=w849, "Decay in"=w851, "AlliGator IV DVR in"=w853) -> ("error out"=w850:errorcluster, "AlliGator IV DVR out"=w852:refnum<data-value>)  [unwired: 4 in, 2 out]
        }
      }
    }
    frame "Decay:Store Cursor-defined Head & Tail Fractions" {
      # "\"Store Cursor-defined Head & Tail Fractions\""
      n228 = Variant To Data(Variant=w859) -> (data=w854:T22, error out=w858:errorcluster)  [unwired: 2 in]
      n229 = call "AlliGator Store Cursor-defined Head & Tail Fractions.vi"("error in (no error)"=w858, "Selected Plot Info"=w854) -> ("Error Out"=w860:errorcluster, "Message"=w856:string)  [unwired: 8 in]
    }
    frame "Decay:Straighten Decay" {
      # "\"Straighten Decay\""
      n230 = Variant To Data(Variant=w877) -> (data=w866:T22, error out=w876:errorcluster)  [unwired: 2 in]
      n231 = call "AlliGator Get Process Plots Indices.vi"("error in (no error)"=w876, "Selected Plot Info"=w866) -> ("error out"=w867:errorcluster, "Selected Plots"=w864:i32[], "Selected Plot Info (dup)"=w865:T22)  [unwired: 7 in]
      n232 = call "XY Graph Straighten Multiple Decays.vi"("error in (no error)"=w867, "Selected Plots"=w864, "Selected Plot Info"=w865) -> ("error out"=w871:errorcluster, "Straightened Plot Message"=w869:string, "Last Straightened Plot"=w872:cluster{"t Array":dbl[], "IRF Array":dbl[]}, "Single Plot?"=w863:bool)  [unwired: 5 in]
      n233 = case shown="True" w863 {
        tunnel: w874 -> [w880 w886]
        tunnel: [w880 w885] -> w873
        tunnel: w872 -> [_ w884]
        tunnel: w871 -> [w879 w883]
        tunnel: [w879 w882] -> w870
        frame False {
        }
        frame True {
          n234 = call "AlliGator IV ROI Decay.vi"("Get (F)/ Set (T)"=TRUE, "error in (no error)"=w883, "Decay in"=w884, "AlliGator IV DVR in"=w886) -> ("error out"=w882:errorcluster, "AlliGator IV DVR out"=w885:refnum<data-value>)  [unwired: 4 in, 2 out]
        }
      }
    }
    frame "Decay:Threshold IRF" {
      # "\"Threshold IRF\""
      n235 = Variant To Data(Variant=w898) -> (data=w887:T22, error out=w897:errorcluster)  [unwired: 2 in]
      n236 = call "AlliGator Thresholded IRF.vi"("error in (no error)"=w897, "Selected Plot Info"=w887) -> ("Error Out"=w892:errorcluster, "Message"=w889:string, "Thresholded IRF"=w893:cluster{"t Array":dbl[], "IRF Array":dbl[]})  [unwired: 7 in]
      n237 = call "AlliGator IV ROI Decay.vi"("Get (F)/ Set (T)"=TRUE, "error in (no error)"=w892, "Decay in"=w893, "AlliGator IV DVR in"=w895) -> ("error out"=w891:errorcluster, "AlliGator IV DVR out"=w894:refnum<data-value>)  [unwired: 4 in, 2 out]
    }
    frame "Decay:Use as Reference Decay" {
      w900 = TRUE ("ON/OFF")
      # "\"Use as Reference Decay\""
      n238 = Unbundle By Name(w914) -> ("Other AlliGator Ctrl Refnums.State Indicators"=w915:refnum<vi>)
      n239 = Variant To Data(Variant=w920) -> (data=w905:T22, error out=w904:errorcluster)  [unwired: 2 in]
      n240 = call "XY Graph Get Selected Plot.vi"("error in (no error)"=w904, "Selected Plot Info"=w905) -> ("error out"=w903:errorcluster, "Plot Name"=w902:string, "Plot"=w901:T29)  [unwired: 4 in, 3 out]
      n241 = call "AlliGator Get-Set State Indicators.vi"("State Indicators Refnum"=w915, "AlliGator State Indicators List"=AlliGator_State_Indicators_List."Reference/IRF Defined", "Error In"=w903, "ON/OFF"=w900, "Set (T)/Get"=w900) -> ("Error Out"=w909:errorcluster)  [unwired: 8 in, 2 out]
      n242 = call "AlliGator IV Reference Decay.vi"("Get (F)/ Set (T)"=TRUE, "Error In"=w909, "Reference Decay Plot Name"=w902, "Reference Decay"=w901, "AlliGator IV DVR in"=w912) -> ("Error Out"=w908:errorcluster, "AlliGator IV DVR out"=w913:refnum<data-value>)  [unwired: 3 in, 2 out]
      n243 = Format Into String(format string="%s: %s", error in=w908, w918, w902) -> (resulting string=w907:string, error out=w917:errorcluster)  [unwired: 1 in]
    }
    frame Default {
      # "\"---- Decays ----\""
    }
  }
  "AlliGator IV DVR out" <- w17
  "error out" <- w6
  "AlliGator Q Elements out" <- w10
  "Script off" <- w7
  n244 = call "AlliGator Package Notebook Messages.vi"("Message Formatting"=w2, "Message"=w3, "AlliGator Q Event in"="AlliGator Q Event in") -> ("[Notebook Message]"=→"[Notebook Message]":T1[])  [unwired: 8 in]
